vi "gums_measureLoop.vi"(0 "File Name":path=path "D:/users/test.dat", 1 "SaveDataQuery":bool=TRUE, 2 "Gain Cluster 2":T3={"Vsd"="Gate", "I 2probe 2"="Gate", "Vxy"="Gate", "Vxx"="Gate", "I leak BG"="Gate", "I leak TG"="Gate", "I Gain 1"=1000000.0, "V Gain 1"=1.0, "conversion factor BG"=1.0, "Vin / Vout 1"=1.0, "V Gain 2"=1.0, "Vin / Vout 2"=1.0, "V Gain 3"=1.0, "Vin / Vout 3"=1.0, "I Gain 2"=1000000.0, "I Gain 3"=1000000.0, "V BG"="Gate", "V TG"="Gate", "conversion factor TG"=1.0, "Vin / Vout 4"=1.0, "Vin / Vout 5"=1.0, "Manual Gain 1"=1.0, "Manual Gain 2"=1.0, "Manual Gain 3"=1.0} {"conversion factor TG" items=["1 V/V"=1.0, "4 V/V"=4.0, "15 V/V"=15.0, "30 V/V"=30.0, "45 V/V"=45.0]; "I Gain 3" items=["1"=1.0, "10"=10.0, "100"=100.0, "1K"=1000.0, "10K"=10000.0, "100K"=100000.0, "1M"=1000000.0, "10M"=10000000.0, "100M"=100000000.0, "1G"=1000000000.0]; "I Gain 2" items=["1"=1.0, "10"=10.0, "100"=100.0, "1K"=1000.0, "10K"=10000.0, "100K"=100000.0, "1M"=1000000.0, "10M"=10000000.0, "100M"=100000000.0, "1G"=1000000000.0]; "V Gain 3" items=["1"=1.0, "10"=10.0, "100"=100.0, "1K"=1000.0, "10K"=10000.0]; "V Gain 2" items=["1"=1.0, "10"=10.0, "100"=100.0, "1K"=1000.0, "10K"=10000.0]; "conversion factor BG" items=["1 V/V"=1.0, "4 V/V"=4.0, "15 V/V"=15.0, "30 V/V"=30.0, "45 V/V"=45.0]; "V Gain 1" items=["1"=1.0, "10"=10.0, "100"=100.0, "1K"=1000.0, "10K"=10000.0]; "I Gain 1" items=["1"=1.0, "10"=10.0, "100"=100.0, "1K"=1000.0, "10K"=10000.0, "100K"=100000.0, "1M"=1000000.0, "10M"=10000000.0, "100M"=100000000.0, "1G"=1000000000.0]}, 3 "Refresh Rate [ms]":i32=1000 min=0, 4 "Device Cluster":T4={"K2400 1"="", "K2400_1"=FALSE, "K2400 2"="", "K2400_2"=FALSE, "Lockin1"="", "Lockin1 present"=FALSE, "Lockin2"="", "Lockin2 present"=FALSE, "TIC"="", "Tcontrol"="OFF", "DMM1"="", "DMM1"=FALSE, "DMM2"="", "DMM2"=FALSE, "DAC"="", "DAC present"=FALSE, "DAC number 1"=0, "Bfield query"=FALSE, "Wvlen query"=FALSE, "ITC signal"={"ITC"=0, "Signal"=enum."Sensor 1"}, "DAC number 2"=0}) -> ()   [LabVIEW 2011]
uses:
  gumLV8p2/D/Labviewsoft/transport/GUMS/Kelvinox drivers/ITCAPPS - Copie.LLB/ITCSignal.ctl
  gumLV8p2/D/Labviewsoft/transport/GUMS/Kelvinox drivers/ITCAPPS - Copie.LLB/ITCSignals.ctl
  stopButton.vi
  DAC/DACreadglobal.vi
  Tglobalvar.vi
  monochromatorcontrol/perHandlemonochromator.vi
  users/nicolas/PHySpec-SDK-1.0.0/Labview-example/libPhyspec/libPhyspec.lvlib
panel:
  out "DAC 2 V [V]":dbl=1916.0
  out "DAC 2 array":dbl[](array[numeric])
  out "DAC number 2":u8=2 min=1 max=8
  out "Formula4Array":dbl[](array[numeric]) format="%.2f"
  out "Formula3Array":dbl[](array[numeric]) format="%.2f"
  out "Formula2Array":dbl[](array[numeric]) format="%.2f"
  in  "Formula 4":string
  in  "Formula 3":string
  in  "Formula 2":string
  out "Formula1Array":dbl[](array[numeric]) format="%.2f"
  in  "Formula 1":string
  out "Rxy Array":dbl[](array[numeric])
  out "ITC signal":T1={"ITC"=0, "Signal"=enum."Sensor 1"}
  in  "Fig3 Y scale 2":string(combo)="0"
  in  "Y-Axis 4":string(combo)="Gate"
  in  "X-Axis 4":string(combo)="Gate"
  out "Isd 4":cluster{"Bg":dbl[], "V_4probe":dbl[]}(graph)
  in  "Fig3 Y scale":string(combo)="0"
  in  "Y-Axis 3":string(combo)="Gate"
  in  "X-Axis 3":string(combo)="Gate"
  in  "Fig1 Y scale":string(combo)="0"
  in  "Fig2 Y scale":string(combo)="0"
  out "Fig 2":cluster{"Bg":dbl[], "V_4probe":dbl[]}(graph)
  in  "Y-Axis 1":string(combo)="Gate"
  in  "X-Axis 1":string(combo)="Gate"
  out "R4probe array":dbl[](array[numeric])
  out "R2probe array":dbl[](array[numeric])
  out "Itg array":dbl[](array[numeric])
  out "Ibg array":dbl[](array[numeric])
  out "Vxy array":dbl[](array[numeric])
  out "Vxx array":dbl[](array[numeric])
  out "Isd array":dbl[](array[numeric])
  out "Vsd array":dbl[](array[numeric])
  out "Vtg array":dbl[](array[numeric])
  out "Vbg array":dbl[](array[numeric])
  out "R 4probe [kOhm]":dbl=1916.0
  out "V_topgate [V]":dbl=1916.0
  out "V_backgate [V]":dbl=1916.0
  out "Vxy [V]":dbl=1916.0
  out "Vxx [V]":dbl=1916.0
  out "R 2probe [kOhm]":dbl=1916.0
  out "I Leak TG[nA]":dbl=1916.0
  out "I Leak BG [nA]":dbl=1916.0
  out "I 2probe [nA]":dbl=1916.0
  out "Vsd [V]":dbl=1916.0
  out "signal cluster":T5
  out "SetIntr Cluster":cluster{dbl, dbl, dbl, dbl, dbl}
  in  "Sensitivity Lockin2":T6(ring)
  in  "Sensitivity Lockin1":T6(ring)
  out "Wavelength array":dbl[](array[numeric])
  out "Wavelength [nm]":dbl=1916.0
  out "Wvlen query":bool
  out "refnum out":refnum<file>
  in  "Y-Axis 2":string(combo)="Gate"
  in  "X-Axis 2":string(combo)="Gate"
  out "DAC number 1":u8=2 min=1 max=8
  out "I K2400 01":dbl[](array[numeric])
  out "I K2400 02":dbl[](array[numeric])
  out "Voltage DMM2":dbl[](array[numeric])
  out "Voltage DMM1":dbl[](array[numeric])
  out "B":dbl[](array[numeric])
  out "Lockin2 X":dbl[](array[numeric])
  out "Lockin2 Y":dbl[](array[numeric])
  out "Lockin1 X":dbl[](array[numeric])
  out "B [T]":dbl=1916.0
  out "T [K]":dbl=1916.0
  out "Bfield query":bool
  out "I K2400_2 [A]":dbl=1916.0
  out "Lockin2 Y [V]":dbl=1916.0
  out "Lockin2 X [V]":dbl=1916.0
  out "V DMM2 [V]":dbl=1916.0
  out "V DMM1 [V]":dbl=1916.0
  out "I K2400_1 [A]":dbl=1916.0
  out "Lockin1 Y [V]":dbl=1916.0
  out "Lockin1 X [V]":dbl=1916.0
  out "Lockin1 Ampl [V]":dbl=1916.0
  out "K2400 1 [V]":dbl=1916.0
  out "K2400 2 [V]":dbl=1916.0
  out "DAC 1 V [V]":dbl=1916.0
  out "DAC present":bool
  out "K2400_2":bool
  out "K2400 2":refnum<visa-resource-name>="GPIB0::11::INSTR"
  out "DAC":refnum<visa-resource-name>="GPIB0::11::INSTR"
  out "DMM2":bool
  out "DMM1":bool
  out "Tcontrol":string
  out "Lockin2 present":bool
  out "Lockin1 present":bool
  out "K2400_1":bool
  out "DMM1":refnum<visa-resource-name>="GPIB0::11::INSTR"
  out "DMM2":refnum<visa-resource-name>="GPIB0::11::INSTR"
  out "TIC":refnum<visa-resource-name>="GPIB0::11::INSTR"
  out "Lockin2":refnum<visa-resource-name>="GPIB0::11::INSTR"
  out "Lockin1":refnum<visa-resource-name>="GPIB0::11::INSTR"
  out "K2400 1":refnum<visa-resource-name>="GPIB0::11::INSTR"
  out "Isd":cluster{"Bg":dbl[], "V_4probe":dbl[]}(graph)
  out "Isd 3":cluster{"Bg":dbl[], "V_4probe":dbl[]}(graph)
  out "stopMainLoop":bool
  out "V K2400_01 array":dbl[](array[numeric])
  out "Lockin1 Y":dbl[](array[numeric])
  out "DAC 1 array":dbl[](array[numeric])
  out "V K2400_02 array":dbl[](array[numeric])
  out "T":dbl[](array[numeric])
  out "Time":dbl[](array[numeric])
  out "Time [s]":dbl=1916.0
  in  "stop":bool
  # "Current run values"
  # "Magnetic Field"
  # "Wavelength"
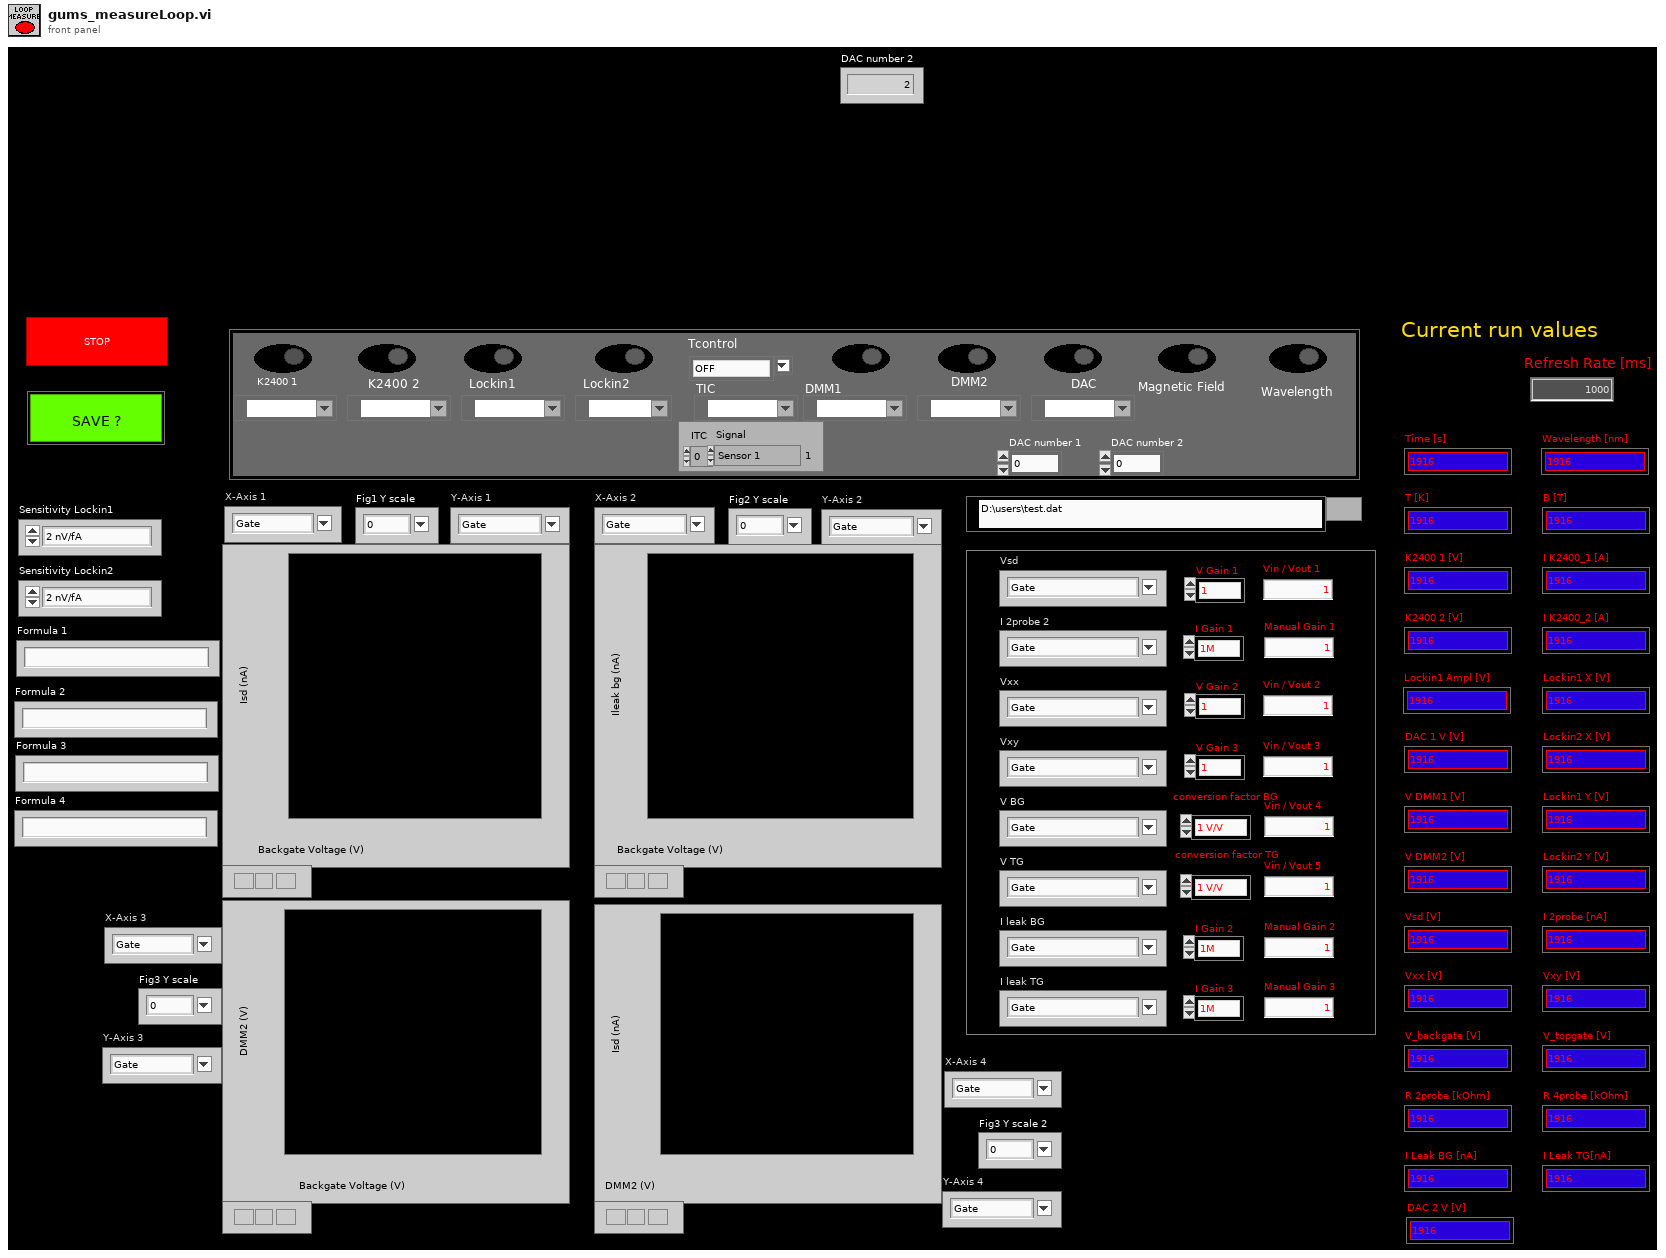
[diagram p1: front panel]
types:
  T1 = typedef "ITCSignal.ctl" = cluster{"ITC":u16, "Signal":T2}
  T2 = typedef "ITCSignals.ctl" = enum16{"Setpoint", "Sensor 1", "Sensor 2", "Sensor 3", "Needle Valve %", "Heater %"}
  T3 = cluster{"Vsd":string, "I 2probe 2":string, "Vxy":string, "Vxx":string, "I leak BG":string, "I leak TG":string, "I Gain 1":dbl, "V Gain 1":dbl, "conversion factor BG":dbl, "Vin / Vout 1":dbl, "V Gain 2":dbl, "Vin / Vout 2":dbl, "V Gain 3":dbl, "Vin / Vout 3":dbl, "I Gain 2":dbl, "I Gain 3":dbl, "V BG":string, "V TG":string, "conversion factor TG":dbl, "Vin / Vout 4":dbl, "Vin / Vout 5":dbl, "Manual Gain 1":dbl, "Manual Gain 2":dbl, "Manual Gain 3":dbl}
  T4 = cluster{"K2400 1":refnum<visa-resource-name>, "K2400_1":bool, "K2400 2":refnum<visa-resource-name>, "K2400_2":bool, "Lockin1":refnum<visa-resource-name>, "Lockin1 present":bool, "Lockin2":refnum<visa-resource-name>, "Lockin2 present":bool, "TIC":refnum<visa-resource-name>, "Tcontrol":string, "DMM1":refnum<visa-resource-name>, "DMM1":bool, "DMM2":refnum<visa-resource-name>, "DMM2":bool, "DAC":refnum<visa-resource-name>, "DAC present":bool, "DAC number 1":u8, "Bfield query":bool, "Wvlen query":bool, "ITC signal":T1, "DAC number 2":u8}
  T5 = cluster{"Output X":dbl, "Output X":dbl, "Voltage output":dbl, "Voltage output":dbl, dbl, dbl}
  T6 = enum16{"2 nV/fA", "5 nV/fA", "10 nV/fA", "20 nV/fA", "50 nV/fA", "100 nV/fA", "200 nV/fA", "500 nV/fA", "1 uV/pA", "2 uV/pA", "5 uV/pA", "10 uV/pA", "20 uV/pA", "50 uV/pA", "100 uV/pA", "200 uV/pA", "500 uV/pA", "1 mV/nA", "2 mV/nA", "5 mV/nA", "10 mV/nA", "20 mV/nA", "50 mV/nA", "100 mV/nA", "200 mV/nA", "500 mV/nA", "1 V/uA"}
  T7 = cluster{"Formula4Array":dbl[], "Formula4Array":dbl[]}
  T8 = cluster{"Output X":dbl, "Output X":dbl, "Voltage output":dbl, "Voltage output":dbl, "I K2400_1 [A]":dbl, "I K2400_2 [A]":dbl}
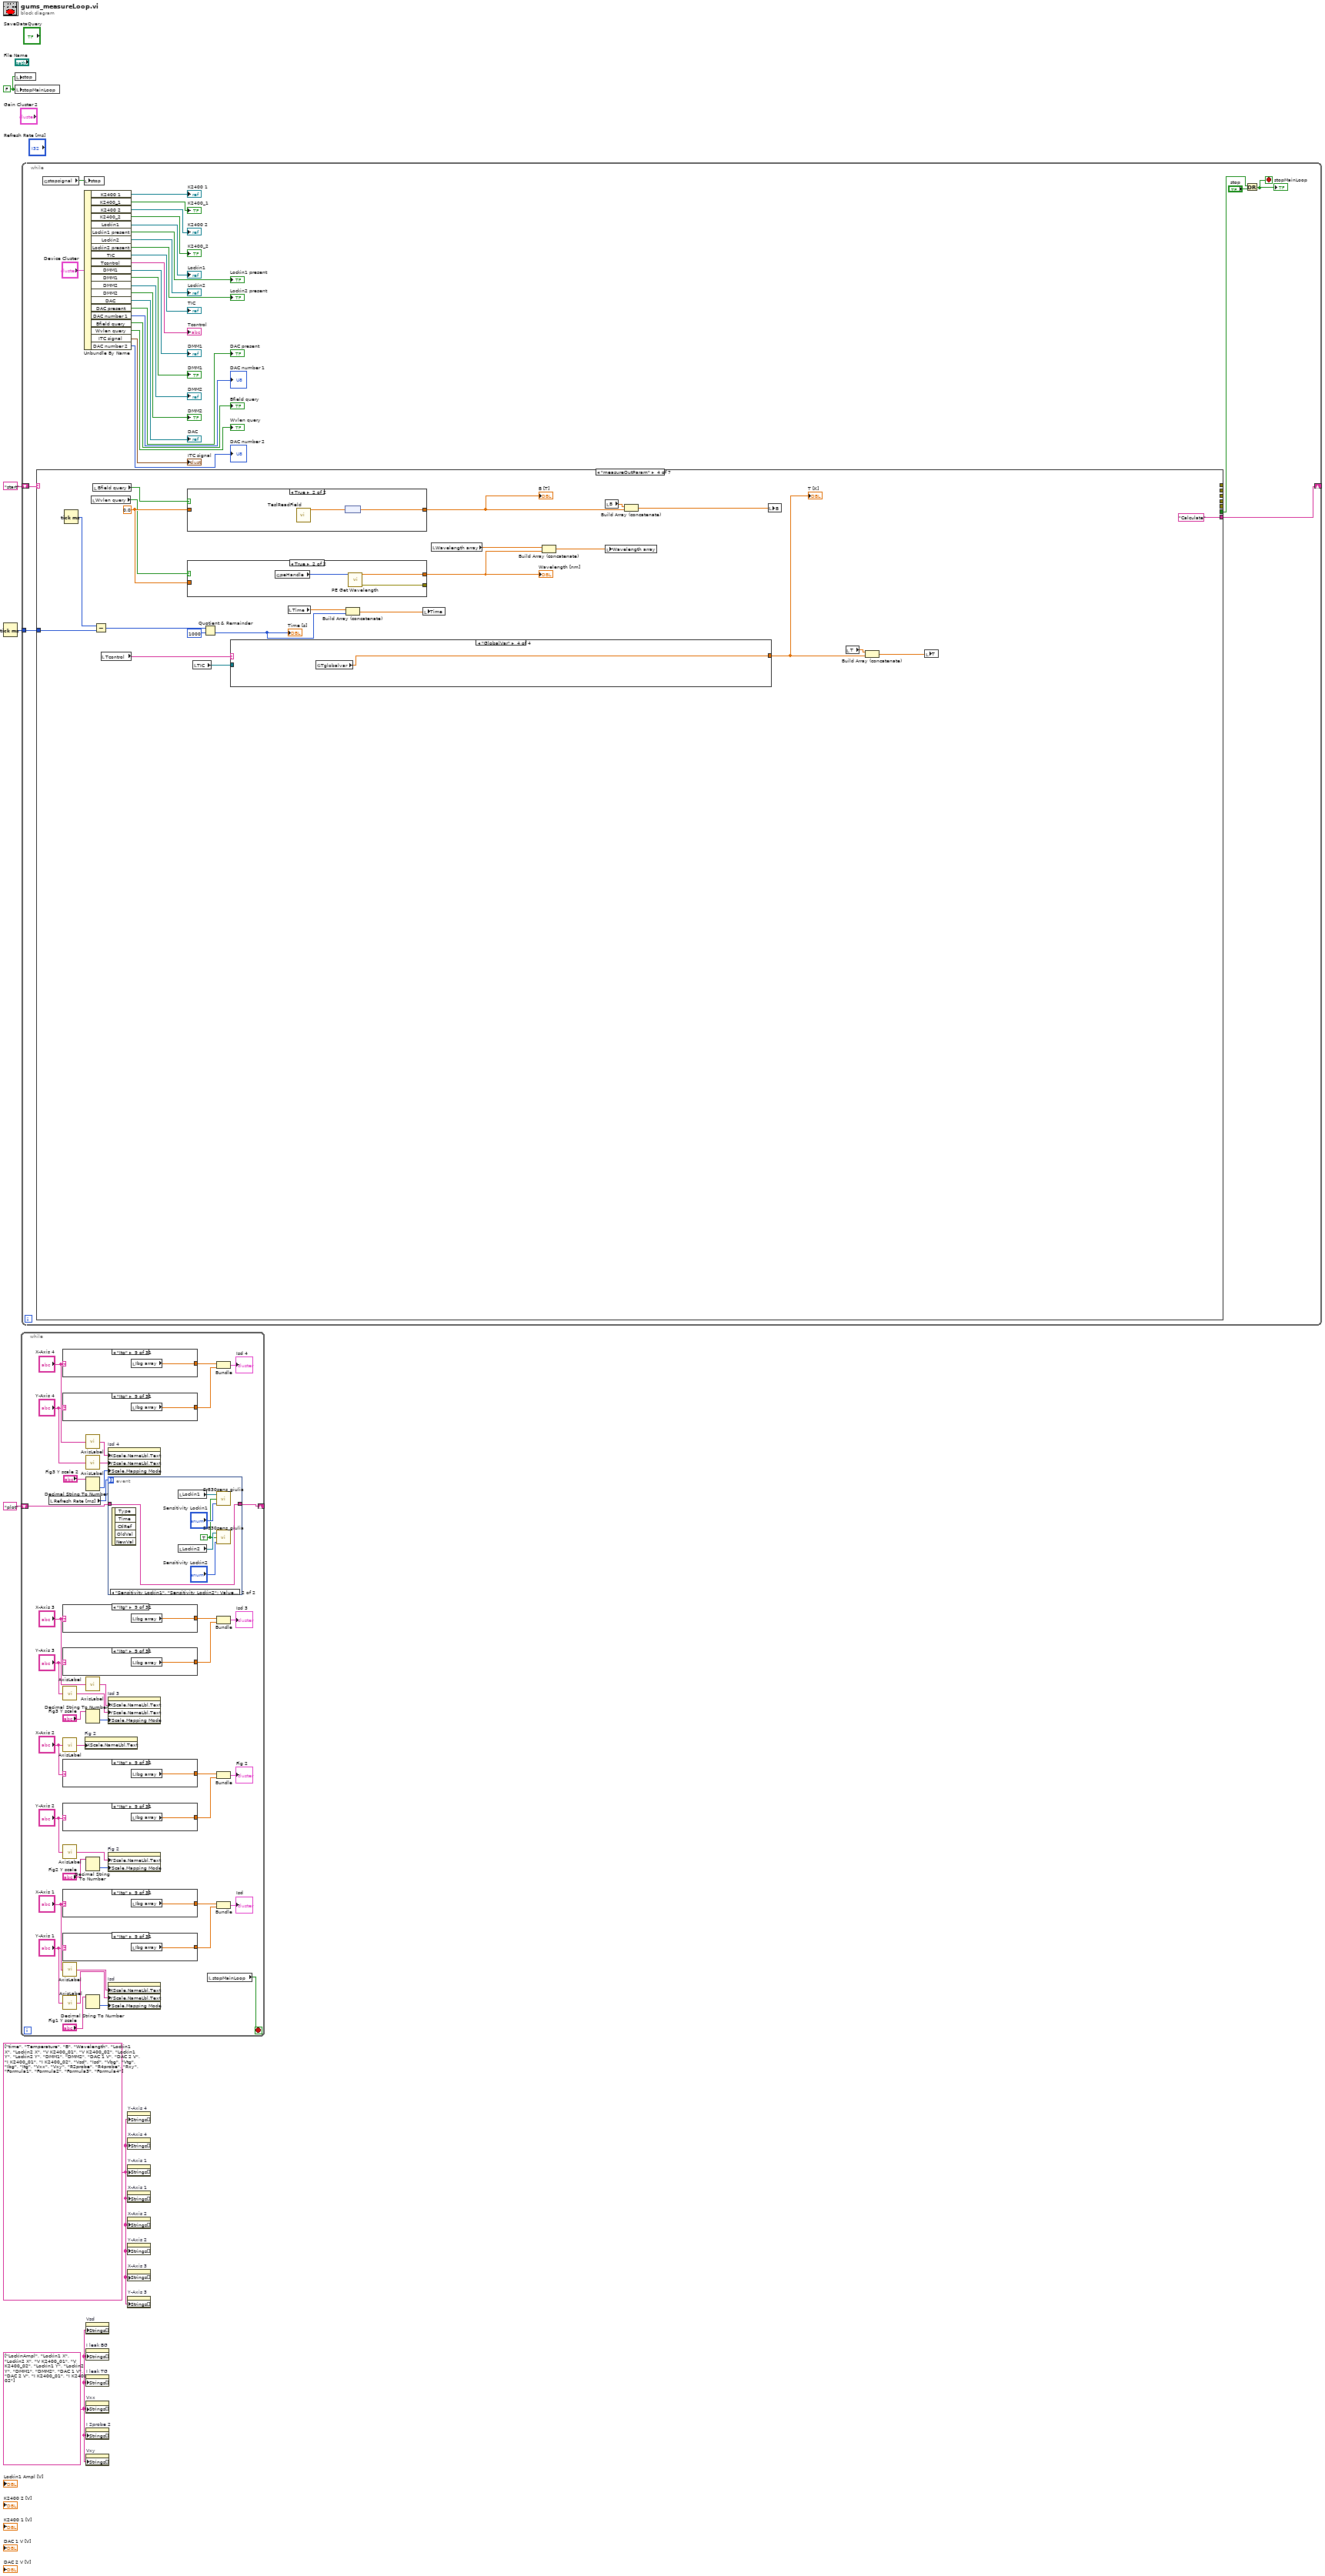
[diagram p0: block diagram]
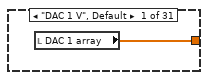
[diagram p2: hidden frame]
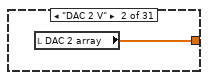
[diagram p3: hidden frame]
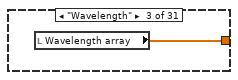
[diagram p4: hidden frame]
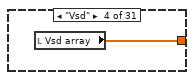
[diagram p5: hidden frame]
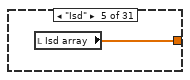
[diagram p6: hidden frame]
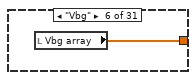
[diagram p7: hidden frame]
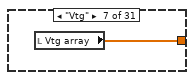
[diagram p8: hidden frame]
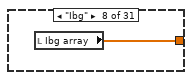
[diagram p9: hidden frame]
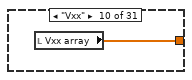
[diagram p10: hidden frame]
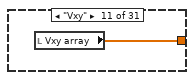
[diagram p11: hidden frame]
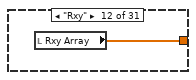
[diagram p12: hidden frame]
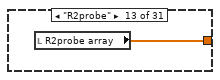
[diagram p13: hidden frame]
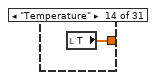
[diagram p14: hidden frame]
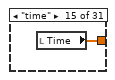
[diagram p15: hidden frame]
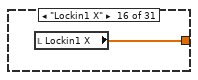
[diagram p16: hidden frame]
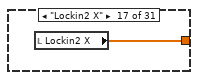
[diagram p17: hidden frame]
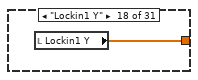
[diagram p18: hidden frame]
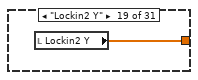
[diagram p19: hidden frame]
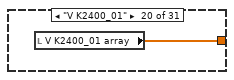
[diagram p20: hidden frame]
diagram:
  w1 = string[] ["time", "Temperature", "B", "Wavelength", "Lockin1 X", "Lockin2 X", "V K2400_01", "V K2400_02", "Lockin1 Y", "Lockin2 Y", "DMM1", "DMM2", "DAC 1 V", "DAC 2 V", "I K2400_01", "I K2400_02", "Vsd", "Isd", "Vbg", "Vtg", "Ibg", "Itg", "Vxx", "Vxy", "R2probe", "R4probe", "Rxy", "Formula1", "Formula2", "Formula3", "Formula4"] ("Axis select")
  w3 = string[] ["LockinAmpl", "Lockin1 X", "Lockin2 X", "V K2400_01", "V K2400_02", "Lockin1 Y", "Lockin2 Y", "DMM1", "DMM2", "DAC 1 V", "DAC 2 V", "I K2400_01", "I K2400_02"] ("Strings []")
  w4 = FALSE ("stop")
  n1 = Tick Count (ms)() -> (millisecond timer value=w5:u32)
  n2 = local write "stop"(w4) -> ()
  n3 = local write "stopMainLoop"(w4) -> ()
  n4 = while {
    shift-right: [w43] -> _
    shift-left: "plot" -> [w44]
    stop <- w45 stop-if-true
    n5 = local read "Refresh Rate [ms]"() -> (w40:i32)
    n6 = case shown="\"Itg\"" "X-Axis 4" {
      tunnel: [w202 w203 w204 w205 w206 w207 w208 w209 w210 w211 w212 w213 w214 w215 w216 w217 w218 w219 w220 w221 w222 w223 w224 w225 w226 w227 w228 w229 w230 w231 w232] -> w18
      frame "DAC 1 V", Default {
        n7 = local read "DAC 1 array"() -> (w202:dbl[])
      }
      frame "DAC 2 V" {
        n8 = local read "DAC 2 array"() -> (w203:dbl[])
      }
      frame "Wavelength" {
        n9 = local read "Wavelength array"() -> (w204:dbl[])
      }
      frame "Vsd" {
        n10 = local read "Vsd array"() -> (w205:dbl[])
      }
      frame "Isd" {
        n11 = local read "Isd array"() -> (w206:dbl[])
      }
      frame "Vbg" {
        n12 = local read "Vbg array"() -> (w207:dbl[])
      }
      frame "Vtg" {
        n13 = local read "Vtg array"() -> (w208:dbl[])
      }
      frame "Ibg" {
        n14 = local read "Ibg array"() -> (w209:dbl[])
      }
      frame "Itg" {
        n15 = local read "Ibg array"() -> (w210:dbl[])
      }
      frame "Vxx" {
        n16 = local read "Vxx array"() -> (w211:dbl[])
      }
      frame "Vxy" {
        n17 = local read "Vxy array"() -> (w212:dbl[])
      }
      frame "Rxy" {
        n18 = local read "Rxy Array"() -> (w213:dbl[])
      }
      frame "R2probe" {
        n19 = local read "R2probe array"() -> (w214:dbl[])
      }
      frame "Temperature" {
        n20 = local read "T"() -> (w215:dbl[])
      }
      frame "time" {
        n21 = local read "Time"() -> (w216:dbl[])
      }
      frame "Lockin1 X" {
        n22 = local read "Lockin1 X"() -> (w217:dbl[])
      }
      frame "Lockin2 X" {
        n23 = local read "Lockin2 X"() -> (w218:dbl[])
      }
      frame "Lockin1 Y" {
        n24 = local read "Lockin1 Y"() -> (w219:dbl[])
      }
      frame "Lockin2 Y" {
        n25 = local read "Lockin2 Y"() -> (w220:dbl[])
      }
      frame "V K2400_01" {
        n26 = local read "V K2400_01 array"() -> (w221:dbl[])
      }
      frame "V K2400_02" {
        n27 = local read "V K2400_02 array"() -> (w222:dbl[])
      }
      frame "I K2400_01" {
        n28 = local read "I K2400 01"() -> (w223:dbl[])
      }
      frame "I K2400_02" {
        n29 = local read "I K2400 02"() -> (w224:dbl[])
      }
      frame "DMM1" {
        n30 = local read "Voltage DMM1"() -> (w225:dbl[])
      }
      frame "DMM2" {
        n31 = local read "Voltage DMM2"() -> (w226:dbl[])
      }
      frame "B" {
        n32 = local read "B"() -> (w227:dbl[])
      }
      frame "R4probe" {
        n33 = local read "R4probe array"() -> (w228:dbl[])
      }
      frame "Formula1" {
        n34 = local read "Formula1Array"() -> (w229:dbl[])
      }
      frame "Formula2" {
        n35 = local read "Formula2Array"() -> (w230:dbl[])
      }
      frame "Formula3" {
        n36 = local read "Formula3Array"() -> (w231:dbl[])
      }
      frame "Formula4" {
        n37 = local read "Formula4Array"() -> (w232:dbl[])
      }
    }
    n38 = case shown="\"Itg\"" "Y-Axis 4" {
      tunnel: [w171 w172 w173 w174 w175 w176 w177 w178 w179 w180 w181 w182 w183 w184 w185 w186 w187 w188 w189 w190 w191 w192 w193 w194 w195 w196 w197 w198 w199 w200 w201] -> w16
      frame "DAC 1 V", Default {
        n39 = local read "DAC 1 array"() -> (w171:dbl[])
      }
      frame "DAC 2 V" {
        n40 = local read "DAC 2 array"() -> (w172:dbl[])
      }
      frame "Wavelength" {
        n41 = local read "Wavelength array"() -> (w173:dbl[])
      }
      frame "Vsd" {
        n42 = local read "Vsd array"() -> (w174:dbl[])
      }
      frame "Isd" {
        n43 = local read "Isd array"() -> (w175:dbl[])
      }
      frame "Vbg" {
        n44 = local read "Vbg array"() -> (w176:dbl[])
      }
      frame "Vtg" {
        n45 = local read "Vtg array"() -> (w177:dbl[])
      }
      frame "Ibg" {
        n46 = local read "Ibg array"() -> (w178:dbl[])
      }
      frame "Itg" {
        n47 = local read "Ibg array"() -> (w179:dbl[])
      }
      frame "Vxx" {
        n48 = local read "Vxx array"() -> (w180:dbl[])
      }
      frame "Vxy" {
        n49 = local read "Vxy array"() -> (w181:dbl[])
      }
      frame "Rxy" {
        n50 = local read "Rxy Array"() -> (w182:dbl[])
      }
      frame "R2probe" {
        n51 = local read "R2probe array"() -> (w183:dbl[])
      }
      frame "Temperature" {
        n52 = local read "T"() -> (w184:dbl[])
      }
      frame "time" {
        n53 = local read "Time"() -> (w185:dbl[])
      }
      frame "Lockin1 X" {
        n54 = local read "Lockin1 X"() -> (w186:dbl[])
      }
      frame "Lockin2 X" {
        n55 = local read "Lockin2 X"() -> (w187:dbl[])
      }
      frame "Lockin1 Y" {
        n56 = local read "Lockin1 Y"() -> (w188:dbl[])
      }
      frame "Lockin2 Y" {
        n57 = local read "Lockin2 Y"() -> (w189:dbl[])
      }
      frame "V K2400_01" {
        n58 = local read "V K2400_01 array"() -> (w190:dbl[])
      }
      frame "V K2400_02" {
        n59 = local read "V K2400_02 array"() -> (w191:dbl[])
      }
      frame "I K2400_01" {
        n60 = local read "I K2400 01"() -> (w192:dbl[])
      }
      frame "I K2400_02" {
        n61 = local read "I K2400 02"() -> (w193:dbl[])
      }
      frame "DMM1" {
        n62 = local read "Voltage DMM1"() -> (w194:dbl[])
      }
      frame "DMM2" {
        n63 = local read "Voltage DMM2"() -> (w195:dbl[])
      }
      frame "B" {
        n64 = local read "B"() -> (w196:dbl[])
      }
      frame "R4probe" {
        n65 = local read "R4probe array"() -> (w197:dbl[])
      }
      frame "Formula1" {
        n66 = local read "Formula1Array"() -> (w198:dbl[])
      }
      frame "Formula2" {
        n67 = local read "Formula2Array"() -> (w199:dbl[])
      }
      frame "Formula3" {
        n68 = local read "Formula3Array"() -> (w200:dbl[])
      }
      frame "Formula4" {
        n69 = local read "Formula4Array"() -> (w201:dbl[])
      }
    }
    n70 = case shown="\"Itg\"" "X-Axis 3" {
      tunnel: [w140 w141 w142 w143 w144 w145 w146 w147 w148 w149 w150 w151 w152 w153 w154 w155 w156 w157 w158 w159 w160 w161 w162 w163 w164 w165 w166 w167 w168 w169 w170] -> w13
      frame "DAC 1 V", Default {
        n71 = local read "DAC 1 array"() -> (w140:dbl[])
      }
      frame "DAC 2 V" {
        n72 = local read "DAC 2 array"() -> (w141:dbl[])
      }
      frame "Wavelength" {
        n73 = local read "Wavelength array"() -> (w142:dbl[])
      }
      frame "Vsd" {
        n74 = local read "Vsd array"() -> (w143:dbl[])
      }
      frame "Isd" {
        n75 = local read "Isd array"() -> (w144:dbl[])
      }
      frame "Vbg" {
        n76 = local read "Vbg array"() -> (w145:dbl[])
      }
      frame "Vtg" {
        n77 = local read "Vtg array"() -> (w146:dbl[])
      }
      frame "Ibg" {
        n78 = local read "Ibg array"() -> (w147:dbl[])
      }
      frame "Itg" {
        n79 = local read "Ibg array"() -> (w148:dbl[])
      }
      frame "Vxx" {
        n80 = local read "Vxx array"() -> (w149:dbl[])
      }
      frame "Vxy" {
        n81 = local read "Vxy array"() -> (w150:dbl[])
      }
      frame "Rxy" {
        n82 = local read "Rxy Array"() -> (w151:dbl[])
      }
      frame "R2probe" {
        n83 = local read "R2probe array"() -> (w152:dbl[])
      }
      frame "Temperature" {
        n84 = local read "T"() -> (w153:dbl[])
      }
      frame "time" {
        n85 = local read "Time"() -> (w154:dbl[])
      }
      frame "Lockin1 X" {
        n86 = local read "Lockin1 X"() -> (w155:dbl[])
      }
      frame "Lockin2 X" {
        n87 = local read "Lockin2 X"() -> (w156:dbl[])
      }
      frame "Lockin1 Y" {
        n88 = local read "Lockin1 Y"() -> (w157:dbl[])
      }
      frame "Lockin2 Y" {
        n89 = local read "Lockin2 Y"() -> (w158:dbl[])
      }
      frame "V K2400_01" {
        n90 = local read "V K2400_01 array"() -> (w159:dbl[])
      }
      frame "V K2400_02" {
        n91 = local read "V K2400_02 array"() -> (w160:dbl[])
      }
      frame "I K2400_01" {
        n92 = local read "I K2400 01"() -> (w161:dbl[])
      }
      frame "I K2400_02" {
        n93 = local read "I K2400 02"() -> (w162:dbl[])
      }
      frame "DMM1" {
        n94 = local read "Voltage DMM1"() -> (w163:dbl[])
      }
      frame "DMM2" {
        n95 = local read "Voltage DMM2"() -> (w164:dbl[])
      }
      frame "B" {
        n96 = local read "B"() -> (w165:dbl[])
      }
      frame "R4probe" {
        n97 = local read "R4probe array"() -> (w166:dbl[])
      }
      frame "Formula1" {
        n98 = local read "Formula1Array"() -> (w167:dbl[])
      }
      frame "Formula2" {
        n99 = local read "Formula2Array"() -> (w168:dbl[])
      }
      frame "Formula3" {
        n100 = local read "Formula3Array"() -> (w169:dbl[])
      }
      frame "Formula4" {
        n101 = local read "Formula4Array"() -> (w170:dbl[])
      }
    }
    n102 = case shown="\"Itg\"" "Y-Axis 3" {
      tunnel: [w109 w110 w111 w112 w113 w114 w115 w116 w117 w118 w119 w120 w121 w122 w123 w124 w125 w126 w127 w128 w129 w130 w131 w132 w133 w134 w135 w136 w137 w138 w139] -> w14
      frame "DAC 1 V", Default {
        n103 = local read "DAC 1 array"() -> (w109:dbl[])
      }
      frame "DAC 2 V" {
        n104 = local read "DAC 2 array"() -> (w110:dbl[])
      }
      frame "Wavelength" {
        n105 = local read "Wavelength array"() -> (w111:dbl[])
      }
      frame "Vsd" {
        n106 = local read "Vsd array"() -> (w112:dbl[])
      }
      frame "Isd" {
        n107 = local read "Isd array"() -> (w113:dbl[])
      }
      frame "Vbg" {
        n108 = local read "Vbg array"() -> (w114:dbl[])
      }
      frame "Vtg" {
        n109 = local read "Vtg array"() -> (w115:dbl[])
      }
      frame "Ibg" {
        n110 = local read "Ibg array"() -> (w116:dbl[])
      }
      frame "Itg" {
        n111 = local read "Ibg array"() -> (w117:dbl[])
      }
      frame "Vxx" {
        n112 = local read "Vxx array"() -> (w118:dbl[])
      }
      frame "Vxy" {
        n113 = local read "Vxy array"() -> (w119:dbl[])
      }
      frame "Rxy" {
        n114 = local read "Rxy Array"() -> (w120:dbl[])
      }
      frame "R2probe" {
        n115 = local read "R2probe array"() -> (w121:dbl[])
      }
      frame "Temperature" {
        n116 = local read "T"() -> (w122:dbl[])
      }
      frame "time" {
        n117 = local read "Time"() -> (w123:dbl[])
      }
      frame "Lockin1 X" {
        n118 = local read "Lockin1 X"() -> (w124:dbl[])
      }
      frame "Lockin2 X" {
        n119 = local read "Lockin2 X"() -> (w125:dbl[])
      }
      frame "Lockin1 Y" {
        n120 = local read "Lockin1 Y"() -> (w126:dbl[])
      }
      frame "Lockin2 Y" {
        n121 = local read "Lockin2 Y"() -> (w127:dbl[])
      }
      frame "V K2400_01" {
        n122 = local read "V K2400_01 array"() -> (w128:dbl[])
      }
      frame "V K2400_02" {
        n123 = local read "V K2400_02 array"() -> (w129:dbl[])
      }
      frame "I K2400_01" {
        n124 = local read "I K2400 01"() -> (w130:dbl[])
      }
      frame "I K2400_02" {
        n125 = local read "I K2400 02"() -> (w131:dbl[])
      }
      frame "DMM1" {
        n126 = local read "Voltage DMM1"() -> (w132:dbl[])
      }
      frame "DMM2" {
        n127 = local read "Voltage DMM2"() -> (w133:dbl[])
      }
      frame "B" {
        n128 = local read "B"() -> (w134:dbl[])
      }
      frame "R4probe" {
        n129 = local read "R4probe array"() -> (w135:dbl[])
      }
      frame "Formula1" {
        n130 = local read "Formula1Array"() -> (w136:dbl[])
      }
      frame "Formula2" {
        n131 = local read "Formula2Array"() -> (w137:dbl[])
      }
      frame "Formula3" {
        n132 = local read "Formula3Array"() -> (w138:dbl[])
      }
      frame "Formula4" {
        n133 = local read "Formula4Array"() -> (w139:dbl[])
      }
    }
    n134 = call "AxisLabel.vi"("Axis"="Y-Axis 3") -> ("X Scale.Name Label.Text"=w29:string)
    n135 = call "AxisLabel.vi"("Axis"="X-Axis 2") -> ("X Scale.Name Label.Text"=w41:string)
    n136 = case shown="\"Itg\"" "X-Axis 2" {
      tunnel: [w47 w48 w49 w50 w51 w52 w53 w54 w55 w56 w57 w58 w59 w60 w61 w62 w63 w64 w65 w66 w67 w68 w69 w70 w71 w72 w73 w74 w75 w76 w77] -> w8
      frame "DAC 1 V", Default {
        n137 = local read "DAC 1 array"() -> (w47:dbl[])
      }
      frame "DAC 2 V" {
        n138 = local read "DAC 2 array"() -> (w48:dbl[])
      }
      frame "Wavelength" {
        n139 = local read "Wavelength array"() -> (w49:dbl[])
      }
      frame "Vsd" {
        n140 = local read "Vsd array"() -> (w50:dbl[])
      }
      frame "Isd" {
        n141 = local read "Isd array"() -> (w51:dbl[])
      }
      frame "Vbg" {
        n142 = local read "Vbg array"() -> (w52:dbl[])
      }
      frame "Vtg" {
        n143 = local read "Vtg array"() -> (w53:dbl[])
      }
      frame "Ibg" {
        n144 = local read "Ibg array"() -> (w54:dbl[])
      }
      frame "Itg" {
        n145 = local read "Ibg array"() -> (w55:dbl[])
      }
      frame "Vxx" {
        n146 = local read "Vxx array"() -> (w56:dbl[])
      }
      frame "Vxy" {
        n147 = local read "Vxy array"() -> (w57:dbl[])
      }
      frame "Rxy" {
        n148 = local read "Rxy Array"() -> (w58:dbl[])
      }
      frame "R2probe" {
        n149 = local read "R2probe array"() -> (w59:dbl[])
      }
      frame "Temperature" {
        n150 = local read "T"() -> (w60:dbl[])
      }
      frame "time" {
        n151 = local read "Time"() -> (w61:dbl[])
      }
      frame "Lockin1 X" {
        n152 = local read "Lockin1 X"() -> (w62:dbl[])
      }
      frame "Lockin2 X" {
        n153 = local read "Lockin2 X"() -> (w63:dbl[])
      }
      frame "Lockin1 Y" {
        n154 = local read "Lockin1 Y"() -> (w64:dbl[])
      }
      frame "Lockin2 Y" {
        n155 = local read "Lockin2 Y"() -> (w65:dbl[])
      }
      frame "V K2400_01" {
        n156 = local read "V K2400_01 array"() -> (w66:dbl[])
      }
      frame "V K2400_02" {
        n157 = local read "V K2400_02 array"() -> (w67:dbl[])
      }
      frame "I K2400_01" {
        n158 = local read "I K2400 01"() -> (w68:dbl[])
      }
      frame "I K2400_02" {
        n159 = local read "I K2400 02"() -> (w69:dbl[])
      }
      frame "DMM1" {
        n160 = local read "Voltage DMM1"() -> (w70:dbl[])
      }
      frame "DMM2" {
        n161 = local read "Voltage DMM2"() -> (w71:dbl[])
      }
      frame "B" {
        n162 = local read "B"() -> (w72:dbl[])
      }
      frame "R4probe" {
        n163 = local read "R4probe array"() -> (w73:dbl[])
      }
      frame "Formula1" {
        n164 = local read "Formula1Array"() -> (w74:dbl[])
      }
      frame "Formula2" {
        n165 = local read "Formula2Array"() -> (w75:dbl[])
      }
      frame "Formula3" {
        n166 = local read "Formula3Array"() -> (w76:dbl[])
      }
      frame "Formula4" {
        n167 = local read "Formula4Array"() -> (w77:dbl[])
      }
    }
    n168 = case shown="\"Itg\"" "Y-Axis 2" {
      tunnel: [w78 w79 w80 w81 w82 w83 w84 w85 w86 w87 w88 w89 w90 w91 w92 w93 w94 w95 w96 w97 w98 w99 w100 w101 w102 w103 w104 w105 w106 w107 w108] -> w9
      frame "DAC 1 V", Default {
        n169 = local read "DAC 1 array"() -> (w78:dbl[])
      }
      frame "DAC 2 V" {
        n170 = local read "DAC 2 array"() -> (w79:dbl[])
      }
      frame "Wavelength" {
        n171 = local read "Wavelength array"() -> (w80:dbl[])
      }
      frame "Vsd" {
        n172 = local read "Vsd array"() -> (w81:dbl[])
      }
      frame "Isd" {
        n173 = local read "Isd array"() -> (w82:dbl[])
      }
      frame "Vbg" {
        n174 = local read "Vbg array"() -> (w83:dbl[])
      }
      frame "Vtg" {
        n175 = local read "Vtg array"() -> (w84:dbl[])
      }
      frame "Ibg" {
        n176 = local read "Ibg array"() -> (w85:dbl[])
      }
      frame "Itg" {
        n177 = local read "Ibg array"() -> (w86:dbl[])
      }
      frame "Vxx" {
        n178 = local read "Vxx array"() -> (w87:dbl[])
      }
      frame "Vxy" {
        n179 = local read "Vxy array"() -> (w88:dbl[])
      }
      frame "Rxy" {
        n180 = local read "Rxy Array"() -> (w89:dbl[])
      }
      frame "R2probe" {
        n181 = local read "R2probe array"() -> (w90:dbl[])
      }
      frame "Temperature" {
        n182 = local read "T"() -> (w91:dbl[])
      }
      frame "time" {
        n183 = local read "Time"() -> (w92:dbl[])
      }
      frame "Lockin1 X" {
        n184 = local read "Lockin1 X"() -> (w93:dbl[])
      }
      frame "Lockin2 X" {
        n185 = local read "Lockin2 X"() -> (w94:dbl[])
      }
      frame "Lockin1 Y" {
        n186 = local read "Lockin1 Y"() -> (w95:dbl[])
      }
      frame "Lockin2 Y" {
        n187 = local read "Lockin2 Y"() -> (w96:dbl[])
      }
      frame "V K2400_01" {
        n188 = local read "V K2400_01 array"() -> (w97:dbl[])
      }
      frame "V K2400_02" {
        n189 = local read "V K2400_02 array"() -> (w98:dbl[])
      }
      frame "I K2400_01" {
        n190 = local read "I K2400 01"() -> (w99:dbl[])
      }
      frame "I K2400_02" {
        n191 = local read "I K2400 02"() -> (w100:dbl[])
      }
      frame "DMM1" {
        n192 = local read "Voltage DMM1"() -> (w101:dbl[])
      }
      frame "DMM2" {
        n193 = local read "Voltage DMM2"() -> (w102:dbl[])
      }
      frame "B" {
        n194 = local read "B"() -> (w103:dbl[])
      }
      frame "R4probe" {
        n195 = local read "R4probe array"() -> (w104:dbl[])
      }
      frame "Formula1" {
        n196 = local read "Formula1Array"() -> (w105:dbl[])
      }
      frame "Formula2" {
        n197 = local read "Formula2Array"() -> (w106:dbl[])
      }
      frame "Formula3" {
        n198 = local read "Formula3Array"() -> (w107:dbl[])
      }
      frame "Formula4" {
        n199 = local read "Formula4Array"() -> (w108:dbl[])
      }
    }
    n200 = call "AxisLabel.vi"("Axis"="Y-Axis 2") -> ("X Scale.Name Label.Text"=w42:string)
    n201 = case shown="\"Itg\"" "X-Axis 1" {
      tunnel: [w264 w265 w266 w267 w268 w269 w270 w271 w272 w273 w274 w275 w276 w277 w278 w279 w280 w281 w282 w283 w284 w285 w286 w287 w288 w289 w290 w291 w292 w293 w294] -> w22
      frame "DAC 1 V", Default {
        n202 = local read "DAC 1 array"() -> (w264:dbl[])
      }
      frame "DAC 2 V" {
        n203 = local read "DAC 2 array"() -> (w265:dbl[])
      }
      frame "Wavelength" {
        n204 = local read "Wavelength array"() -> (w266:dbl[])
      }
      frame "Vsd" {
        n205 = local read "Vsd array"() -> (w267:dbl[])
      }
      frame "Isd" {
        n206 = local read "Isd array"() -> (w268:dbl[])
      }
      frame "Vbg" {
        n207 = local read "Vbg array"() -> (w269:dbl[])
      }
      frame "Vtg" {
        n208 = local read "Vtg array"() -> (w270:dbl[])
      }
      frame "Ibg" {
        n209 = local read "Ibg array"() -> (w271:dbl[])
      }
      frame "Itg" {
        n210 = local read "Ibg array"() -> (w272:dbl[])
      }
      frame "Vxx" {
        n211 = local read "Vxx array"() -> (w273:dbl[])
      }
      frame "Vxy" {
        n212 = local read "Vxy array"() -> (w274:dbl[])
      }
      frame "Rxy" {
        n213 = local read "Rxy Array"() -> (w275:dbl[])
      }
      frame "R2probe" {
        n214 = local read "R2probe array"() -> (w276:dbl[])
      }
      frame "Temperature" {
        n215 = local read "T"() -> (w277:dbl[])
      }
      frame "time" {
        n216 = local read "Time"() -> (w278:dbl[])
      }
      frame "Lockin1 X" {
        n217 = local read "Lockin1 X"() -> (w279:dbl[])
      }
      frame "Lockin2 X" {
        n218 = local read "Lockin2 X"() -> (w280:dbl[])
      }
      frame "Lockin1 Y" {
        n219 = local read "Lockin1 Y"() -> (w281:dbl[])
      }
      frame "Lockin2 Y" {
        n220 = local read "Lockin2 Y"() -> (w282:dbl[])
      }
      frame "V K2400_01" {
        n221 = local read "V K2400_01 array"() -> (w283:dbl[])
      }
      frame "V K2400_02" {
        n222 = local read "V K2400_02 array"() -> (w284:dbl[])
      }
      frame "I K2400_01" {
        n223 = local read "I K2400 01"() -> (w285:dbl[])
      }
      frame "I K2400_02" {
        n224 = local read "I K2400 02"() -> (w286:dbl[])
      }
      frame "DMM1" {
        n225 = local read "Voltage DMM1"() -> (w287:dbl[])
      }
      frame "DMM2" {
        n226 = local read "Voltage DMM2"() -> (w288:dbl[])
      }
      frame "B" {
        n227 = local read "B"() -> (w289:dbl[])
      }
      frame "R4probe" {
        n228 = local read "R4probe array"() -> (w290:dbl[])
      }
      frame "Formula1" {
        n229 = local read "Formula1Array"() -> (w291:dbl[])
      }
      frame "Formula2" {
        n230 = local read "Formula2Array"() -> (w292:dbl[])
      }
      frame "Formula3" {
        n231 = local read "Formula3Array"() -> (w293:dbl[])
      }
      frame "Formula4" {
        n232 = local read "Formula4Array"() -> (w294:dbl[])
      }
    }
    n233 = case shown="\"Itg\"" "Y-Axis 1" {
      tunnel: [w233 w234 w235 w236 w237 w238 w239 w240 w241 w242 w243 w244 w245 w246 w247 w248 w249 w250 w251 w252 w253 w254 w255 w256 w257 w258 w259 w260 w261 w262 w263] -> w19
      frame "DAC 1 V", Default {
        n234 = local read "DAC 1 array"() -> (w233:dbl[])
      }
      frame "DAC 2 V" {
        n235 = local read "DAC 2 array"() -> (w234:dbl[])
      }
      frame "Wavelength" {
        n236 = local read "Wavelength array"() -> (w235:dbl[])
      }
      frame "Vsd" {
        n237 = local read "Vsd array"() -> (w236:dbl[])
      }
      frame "Isd" {
        n238 = local read "Isd array"() -> (w237:dbl[])
      }
      frame "Vbg" {
        n239 = local read "Vbg array"() -> (w238:dbl[])
      }
      frame "Vtg" {
        n240 = local read "Vtg array"() -> (w239:dbl[])
      }
      frame "Ibg" {
        n241 = local read "Ibg array"() -> (w240:dbl[])
      }
      frame "Itg" {
        n242 = local read "Ibg array"() -> (w241:dbl[])
      }
      frame "Vxx" {
        n243 = local read "Vxx array"() -> (w242:dbl[])
      }
      frame "Vxy" {
        n244 = local read "Vxy array"() -> (w243:dbl[])
      }
      frame "Rxy" {
        n245 = local read "Rxy Array"() -> (w244:dbl[])
      }
      frame "R2probe" {
        n246 = local read "R2probe array"() -> (w245:dbl[])
      }
      frame "Temperature" {
        n247 = local read "T"() -> (w246:dbl[])
      }
      frame "time" {
        n248 = local read "Time"() -> (w247:dbl[])
      }
      frame "Lockin1 X" {
        n249 = local read "Lockin1 X"() -> (w248:dbl[])
      }
      frame "Lockin2 X" {
        n250 = local read "Lockin2 X"() -> (w249:dbl[])
      }
      frame "Lockin1 Y" {
        n251 = local read "Lockin1 Y"() -> (w250:dbl[])
      }
      frame "Lockin2 Y" {
        n252 = local read "Lockin2 Y"() -> (w251:dbl[])
      }
      frame "V K2400_01" {
        n253 = local read "V K2400_01 array"() -> (w252:dbl[])
      }
      frame "V K2400_02" {
        n254 = local read "V K2400_02 array"() -> (w253:dbl[])
      }
      frame "I K2400_01" {
        n255 = local read "I K2400 01"() -> (w254:dbl[])
      }
      frame "I K2400_02" {
        n256 = local read "I K2400 02"() -> (w255:dbl[])
      }
      frame "DMM1" {
        n257 = local read "Voltage DMM1"() -> (w256:dbl[])
      }
      frame "DMM2" {
        n258 = local read "Voltage DMM2"() -> (w257:dbl[])
      }
      frame "B" {
        n259 = local read "B"() -> (w258:dbl[])
      }
      frame "R4probe" {
        n260 = local read "R4probe array"() -> (w259:dbl[])
      }
      frame "Formula1" {
        n261 = local read "Formula1Array"() -> (w260:dbl[])
      }
      frame "Formula2" {
        n262 = local read "Formula2Array"() -> (w261:dbl[])
      }
      frame "Formula3" {
        n263 = local read "Formula3Array"() -> (w262:dbl[])
      }
      frame "Formula4" {
        n264 = local read "Formula4Array"() -> (w263:dbl[])
      }
    }
    n265 = call "AxisLabel.vi"("Axis"="X-Axis 1") -> ("X Scale.Name Label.Text"=w38:string)
    n266 = call "AxisLabel.vi"("Axis"="Y-Axis 1") -> ("X Scale.Name Label.Text"=w37:string)
    n267 = property on="Fig 2" class="XYGraph (strict)"("XScale.NameLbl.Text"=w41) -> ()  [unwired: 2 in, 2 out]
    n268 = call "AxisLabel.vi"("Axis"="X-Axis 4") -> ("X Scale.Name Label.Text"=w24:string)
    n269 = call "AxisLabel.vi"("Axis"="Y-Axis 4") -> ("X Scale.Name Label.Text"=w25:string)
    n270 = Decimal String To Number(string="Fig3 Y scale 2") -> (number=w23:i32)  [unwired: 2 in, 1 out]
    n271 = call "AxisLabel.vi"("Axis"="X-Axis 3") -> ("X Scale.Name Label.Text"=w30:string)
    n272 = Decimal String To Number(string="Fig3 Y scale") -> (number=w28:i32)  [unwired: 2 in, 1 out]
    n273 = Decimal String To Number(string="Fig2 Y scale") -> (number=w34:i32)  [unwired: 2 in, 1 out]
    n274 = Decimal String To Number(string="Fig1 Y scale") -> (number=w32:i32)  [unwired: 2 in, 1 out]
    n275 = property on="Isd 4" class="XYGraph (strict)"("XScale.NameLbl.Text"=w24, "YScale.NameLbl.Text"=w25, "YScale.Mapping Mode"=w23) -> ()  [unwired: 2 in, 2 out]
    n276 = event shown="[1] \"Sensitivity Lockin1\", \"Sensitivity Lockin2\": Value Change" {
      selector: _ -> [_ _]
      dyn-events: _ -> [_ _]
      timeout: w40 -> [_ _]
      tunnel: w44 -> [w295 w296]
      tunnel: [w295 w296] -> w43
      event Timeout {
        n277 = event-data() -> ()  [unwired: 1 in, 2 out]
      }
      event "Sensitivity Lockin1", "Sensitivity Lockin2": Value Change {
        w297 = TRUE ("Change sensitivity ?")
        n278 = event-data() -> ()  [unwired: 1 in, 5 out]
        n279 = local read "Lockin1"() -> (w301:refnum<visa-resource-name>)
        n280 = local read "Lockin2"() -> (w300:refnum<visa-resource-name>)
        n281 = call "Sr830sens_giulia.vi"("Sr 830 sensitivity"="Sensitivity Lockin1", "Change sensitivity ?"=w297, "SR830"=w301) -> ()  [unwired: 1 out]
        n282 = call "Sr830sens_giulia.vi"("Sr 830 sensitivity"="Sensitivity Lockin2", "Change sensitivity ?"=w297, "SR830"=w300) -> ()  [unwired: 1 out]
      }
    }
    n283 = property on="Isd 3" class="XYGraph (strict)"("XScale.NameLbl.Text"=w30, "YScale.NameLbl.Text"=w29, "YScale.Mapping Mode"=w28) -> ()  [unwired: 2 in, 2 out]
    n284 = property on="Fig 2" class="XYGraph (strict)"("YScale.NameLbl.Text"=w42, "YScale.Mapping Mode"=w34) -> ()  [unwired: 2 in, 2 out]
    n285 = property on="Isd" class="XYGraph (strict)"("XScale.NameLbl.Text"=w38, "YScale.NameLbl.Text"=w37, "YScale.Mapping Mode"=w32) -> ()  [unwired: 2 in, 2 out]
    n286 = local read "stopMainLoop"() -> (w45:bool)
    n287 = Bundle("Formula4Array"=w18, "Formula4Array"=w16) -> (→"Isd 4":T7)  [unwired: 1 out]
    n288 = Bundle("Formula4Array"=w13, "Formula4Array"=w14) -> (→"Isd 3":T7)  [unwired: 1 out]
    n289 = Bundle("Formula4Array"=w8, "Formula4Array"=w9) -> (→"Fig 2":T7)  [unwired: 1 out]
    n290 = Bundle("Formula4Array"=w22, "Formula4Array"=w19) -> (→"Isd":T7)  [unwired: 1 out]
  }
  n291 = while {
    shift-right: [w329] -> _
    shift-left: "start" -> [w330]
    tunnel: w5 -> [w326]
    stop <- w325 stop-if-true
    n292 = case shown="\"measureOutParam\"" w330 {
      tunnel: ["measureSetInstruments" "measureSignal" "measureOutParam" "Calculate" "measureSetInstruments" "writeFile" ""] -> w329
      tunnel: [_ _ _ _ _ _ TRUE ("x")] -> w327
      tunnel: w326 -> [_ _ _ w558 _ _ _]
      tunnel: [_ _ _ _ w580 _ _] -> _
      tunnel: [_ _ _ _ _ w666 _] -> _
      tunnel: [_ _ _ _ _ w656 _] -> _
      tunnel: [_ _ _ _ _ w655 _] -> _
      tunnel: [_ _ _ _ _ w654 _] -> _
      frame "start", Default {
        w339 = "\t"
        w346 = "\t"
        w354 = "\t"
        w335 = "\t"
        w361 = "\t"
        w355 = "\t"
        w370 = "\t"
        # "Time\nT\nB\nWavelength\nDAC\nV K2400_01\nV K2400_02\nLockin V\nDMM1\nDMM2\nLK 1 X\nLK 1 Y\nLK2 X\nLK2 Y\nI K2400_01\nI K2400_02\nVsd\nVbgate\nVtopgate\nI2probe\nIleak bg\nIleak tg\nVxx\nVxy\nR2probe\nR4probe"
        n293 = Initialize Array(0) -> (→"Time" →"T" →"DAC 1 array" →"V K2400_01 array" →"V K2400_02 array" →"Lockin1 Y" →"Lockin1 X" →"Lockin2 Y" →"Lockin2 X" →"B" →"Voltage DMM1" →"Voltage DMM2" →"I K2400 02" →"I K2400 01" →"Wavelength array" →"Vbg array" →"Vtg array" →"Vsd array" →"Isd array" →"Vxx array" →"Vxy array" →"Ibg array" →"Itg array" →"R2probe array" →"R4probe array" →"Rxy Array" →"DAC 2 array":i32[])  [unwired: 1 out]
        n294 = Get Date/Time In Seconds() -> (seconds since 1Jan1904=w384:timestamp)
        n295 = Concatenate Strings("I 2probe [nA]" ("string"), w346, "Ileak bg [nA]" ("string"), w346, "Ileak tg [nA]" ("string"), w346) -> (w344:string)
        n296 = Get Date/Time String(date format (0)=1, seconds (now)=w384) -> (date string=w381:string, time string=w382:string)  [unwired: 1 out]
        n297 = Concatenate Strings("Vxx [V]" ("string"), w339, "Vxy [V]" ("string"), w339, "R2probe [kOhm]" ("string"), w339, "R4probe [kOhm]" ("string")) -> (w338:string)
        n298 = Concatenate Strings(w382, "\t", w381, "\r\n") -> (w377:string)
        n299 = Concatenate Strings("DMM1 [V]" ("string"), w361, "DMM2 [V]" ("string"), w361, "Lockin1 X [V]" ("string"), w361, "Lockin1 Y [V]" ("string"), w361, "Lockin2 X [V]" ("string"), w361, "Lockin2 Y [V]" ("string"), w361) -> (w357:string)
        n300 = Concatenate Strings("DAC 1 [V]" ("string"), w335, "DAC 2 [V]" ("string"), w335, "K2400_01 [V]" ("string"), w335, "K2400_02 [V]" ("string"), w335, "Lockin V [V]" ("string"), w335) -> (w358:string)
        n301 = Concatenate Strings("Time [s]", w370, "T [K]" ("chaîne"), w370, "B [T]" ("chaîne"), w370, "Wavelength [nm]" ("chaîne"), w370) -> (w376:string)
        n302 = Concatenate Strings("Vsd [V]" ("string"), w354, "Vbg [V]" ("string"), w354, "Vtg [V]" ("string"), w354) -> (w350:string)
        n303 = Concatenate Strings("I K2400_01 [A]" ("string"), w355, "I K2400_02 [A]" ("string"), w355) -> (w356:string)
        n304 = local read "File Name"() -> (w388:path)
        n305 = Concatenate Strings(w377, w376, w358, w357, w356, w350, w344, w338, "\r\n") -> (w378:string)
        n306 = Open/Create/Replace File(file path (use dialog)=w388, prompt="Enter data filename", operation (0:open)=5) -> (refnum out=w385:refnum<file>, error out=w374:errorcluster)  [unwired: 1 in, 3 out]
        n307 = Write to Text File(file (use dialog)=w385, text=w378, error in=w374) -> (refnum out=→"refnum out":refnum<file>, error out=w337:errorcluster)  [unwired: 2 out]
        n308 = case shown="No Error" w337 {
          frame No Error {
          }
          frame Error {
          }
        }
      }
      frame "measureSetInstruments" {
        w403 = errorcluster {"status"=FALSE, "code"=0, "source"=""} ("error in (no error)")
        w398 = 0.0
        n309 = local read "K2400_1"() -> (w421:bool)
        n310 = local read "K2400_2"() -> (w420:bool)
        n311 = local read "K2400 1"() -> (w413:refnum<visa-resource-name>)
        n312 = local read "K2400 2"() -> (w412:refnum<visa-resource-name>)
        n313 = local read "Lockin1 present"() -> (w410:bool)
        n314 = local read "Lockin1"() -> (w411:refnum<visa-resource-name>)
        n315 = case shown="True" w421 {
          tunnel: [w459 w464] -> w407
          tunnel: w398 -> [w459 _]
          tunnel: w413 -> [_ w463]
          tunnel: w403 -> [_ _]
          tunnel: [w459 w460] -> w402
          frame False {
          }
          frame True {
            n316 = call "K2400_write&read.vi"("Command"="READ?", "VISA Resource Name"=w463) -> ("error out"=w462:errorcluster, "Read"=w468:string)  [unwired: 1 in]
            n317 = case shown="No Error" w462 {
              frame No Error {
              }
              frame Error {
              }
            }
            n318 = Match Pattern(string=w468, regular expression=",") -> (before substring=w465:string, after substring=w461:string)  [unwired: 3 out]
            n319 = Fract/Exp String To Number(string=w465) -> (number=w464:dbl)  [unwired: 4 out]
            n320 = Fract/Exp String To Number(string=w461) -> (number=w460:dbl)  [unwired: 4 out]
          }
        }
        "I K2400_1 [A]" <- w402
        n321 = case shown="True" w420 {
          tunnel: [w448 w454] -> w405
          tunnel: w398 -> [w448 _]
          tunnel: w412 -> [_ w453]
          tunnel: w403 -> [_ w452]
          tunnel: [w448 w449] -> w401
          frame False {
          }
          frame True {
            n322 = call "K2400_write&read.vi"("error in (no error)"=w452, "Command"="READ?", "VISA Resource Name"=w453) -> ("error out"=w451:errorcluster, "Read"=w458:string)
            n323 = case shown="No Error" w451 {
              frame No Error {
              }
              frame Error {
              }
            }
            n324 = Match Pattern(string=w458, regular expression=",") -> (before substring=w455:string, after substring=w450:string)  [unwired: 3 out]
            n325 = Fract/Exp String To Number(string=w455) -> (number=w454:dbl)  [unwired: 4 out]
            n326 = Fract/Exp String To Number(string=w450) -> (number=w449:dbl)  [unwired: 4 out]
          }
        }
        "I K2400_2 [A]" <- w401
        n327 = global read "DACreadglobal.vi" "DAC read global (mV)"() -> (w392:dbl[])
        n328 = local read "DAC number 1"() -> (w409:u8)
        n329 = local read "DAC present"() -> (w395:bool)
        n330 = case shown="True" w410 {
          tunnel: [w430 w432] -> w406
          tunnel: w398 -> [w430 _]
          tunnel: w411 -> [_ w431]
          frame False {
          }
          frame True {
            n331 = VISA Write(VISA resource name=w431, write buffer="SLVL? " ("chaîne")) -> (VISA resource name out=w436:refnum<visa-resource-name>, error out=w435:errorcluster)  [unwired: 1 in, 1 out]
            n332 = VISA Read(VISA resource name=w436, byte count=u32 1024, error in (no error)=w435) -> (read buffer=w433:string)  [unwired: 3 out]
            n333 = Fract/Exp String To Number(string=w433) -> (number=w432:dbl)  [unwired: 4 out]
          }
        }
        n334 = local read "DAC"() -> (w399:refnum<visa-resource-name>)
        n335 = case shown="True" w395 {
          selector: w395 -> [w439 w445]
          tunnel: [w440 w446] -> w408
          tunnel: w398 -> [w440 _]
          tunnel: w399 -> [_ _]
          tunnel: w409 -> [_ w444]
          tunnel: [w439 w445] -> w393
          tunnel: w392 -> [w438 w441]
          tunnel: [w438 w441] -> w391
          frame False {
          }
          frame True {
            n336 = Decrement(x=w444) -> (x-1=w443:u8)
            n337 = Index Array(array=w441, index=w443) -> (element=w442:dbl)
            n338 = Divide(x=w442, y=1000.0) -> (x/y=w446:dbl)
          }
        }
        n339 = local read "DAC number 2"() -> (w400:u8)
        n340 = local read "DAC 1 array"() -> (w419:dbl[])
        n341 = local read "V K2400_01 array"() -> (w416:dbl[])
        n342 = local read "V K2400_02 array"() -> (w417:dbl[])
        n343 = local write "Lockin1 Ampl [V]"(w406) -> ()
        n344 = case shown="True" w393 {
          tunnel: [w423 w428] -> w394
          tunnel: w398 -> [w423 _]
          tunnel: w399 -> [_ _]
          tunnel: w400 -> [_ w425]
          tunnel: w391 -> [_ w426]
          frame False {
          }
          frame True {
            n345 = Decrement(x=w425) -> (x-1=w427:u8)
            n346 = Index Array(array=w426, index=w427) -> (element=w424:dbl)
            n347 = Divide(x=w424, y=1000.0) -> (x/y=w428:dbl)
          }
        }
        n348 = local write "DAC 1 V [V]"(w408) -> ()
        n349 = Build Array (concatenate)(w419, w408) -> (w418:dbl[])
        n350 = local write "K2400 1 [V]"(w407) -> ()
        n351 = local write "K2400 2 [V]"(w405) -> ()
        n352 = local write "DAC 1 array"(w418) -> ()
        n353 = Build Array (concatenate)(w416, w407) -> (w414:dbl[])
        n354 = Build Array (concatenate)(w417, w405) -> (w415:dbl[])
        n355 = local write "V K2400_01 array"(w414) -> ()
        n356 = local write "V K2400_02 array"(w415) -> ()
        n357 = local read "DAC 2 array"() -> (w397:dbl[])
        n358 = local write "DAC 2 V [V]"(w394) -> ()
        n359 = Bundle(w408, w407, w405, w406, w394) -> (→"SetIntr Cluster":cluster{dbl, dbl, dbl, dbl, dbl})  [unwired: 1 in]
        n360 = Build Array (concatenate)(w397, w394) -> (w396:dbl[])
        n361 = local write "DAC 2 array"(w396) -> ()
      }
      frame "measureSignal" {
        w500 = 0.0
        n362 = local read "K2400_1"() -> (w511:bool)
        n363 = local read "K2400 1"() -> (w512:refnum<visa-resource-name>)
        n364 = local read "DMM1"() -> (w507:bool)
        n365 = local read "DMM1"() -> (w508:refnum<visa-resource-name>)
        n366 = local read "Lockin1 present"() -> (w509:bool)
        n367 = local read "Lockin1"() -> (w510:refnum<visa-resource-name>)
        n368 = case shown="True" w507 {
          tunnel: w508 -> [_ w529]
          tunnel: [w525 w528] -> w473
          tunnel: w500 -> [w525 w527]
          tunnel: [w525 w527] -> w476
          frame False {
          }
          frame True {
            n369 = call "AGILENT34401a_read.vi"("VISA Resource Name in"=w529) -> ("Voltage output"=w528:dbl, "error out"=w526:errorcluster)  [unwired: 1 out]
            n370 = case shown="No Error" w526 {
              frame No Error {
              }
              frame Error {
              }
            }
          }
        }
        "V DMM1 [V]" <- w473
        n371 = case shown="False" w511 {
          tunnel: [w531 w532] -> w471
          tunnel: w512 -> [_ _]
          tunnel: w500 -> [w531 _]
          tunnel: "READ?" -> [w530 w533]
          tunnel: [w530 w533] -> w478
          frame False {
          }
          frame True {
            n372 = local read "I K2400_1 [A]"() -> (w532:dbl)
          }
        }
        n373 = case shown="True" w509 {
          tunnel: w510 -> [_ w540]
          tunnel: [w534 w539] -> w475
          tunnel: [w534 w538] -> w488
          tunnel: w500 -> [w534 w536]
          tunnel: [w535 w537] -> w480
          tunnel: "1,4" ("Variable") -> [w535 w537]
          tunnel: [w534 w536] -> w477
          frame False {
          }
          frame True {
            n374 = call "Lockin_SR830_readXY.vi"("Variable"=w537, "VISA Resource Name"=w540) -> ("Output Y"=w538:dbl, "Output X"=w539:dbl)
          }
        }
        "Lockin1 X [V]" <- w475
        "Lockin1 Y [V]" <- w488
        n375 = local read "I K2400 01"() -> (w499:dbl[])
        n376 = local read "K2400_2"() -> (w501:bool)
        n377 = local read "K2400 2"() -> (w502:refnum<visa-resource-name>)
        n378 = local read "Lockin2 present"() -> (w503:bool)
        n379 = local read "Lockin1 Y"() -> (w489:dbl[])
        n380 = local read "Lockin1 X"() -> (w492:dbl[])
        n381 = local read "Lockin2"() -> (w504:refnum<visa-resource-name>)
        n382 = case shown="False" w501 {
          tunnel: [w514 w515] -> w469
          tunnel: w502 -> [_ _]
          tunnel: w500 -> [w514 _]
          tunnel: w478 -> [_ _]
          frame False {
          }
          frame True {
            n383 = local read "I K2400_2 [A]"() -> (w515:dbl)
          }
        }
        n384 = Build Array (concatenate)(w499, w471) -> (w498:dbl[])
        n385 = local read "Voltage DMM1"() -> (w484:dbl[])
        n386 = local read "DMM2"() -> (w506:bool)
        n387 = local read "DMM2"() -> (w505:refnum<visa-resource-name>)
        n388 = case shown="True" w503 {
          tunnel: w504 -> [_ w520]
          tunnel: [w516 w519] -> w474
          tunnel: [w516 w518] -> w494
          tunnel: w477 -> [w516 _]
          tunnel: w480 -> [_ w517]
          frame False {
          }
          frame True {
            n389 = call "Lockin_SR830_readXY.vi"("Variable"=w517, "VISA Resource Name"=w520) -> ("Output Y"=w518:dbl, "Output X"=w519:dbl)
          }
        }
        "Lockin2 X [V]" <- w474
        "Lockin2 Y [V]" <- w494
        n390 = local write "I K2400 01"(w498) -> ()
        n391 = Build Array (concatenate)(w489, w488) -> (w490:dbl[])
        n392 = Build Array (concatenate)(w492, w475) -> (w491:dbl[])
        n393 = case shown="True" w506 {
          tunnel: w505 -> [_ w524]
          tunnel: [w521 w523] -> w472
          tunnel: w476 -> [w521 _]
          frame False {
          }
          frame True {
            n394 = call "AGILENT34401a_read.vi"("VISA Resource Name in"=w524) -> ("Voltage output"=w523:dbl, "error out"=w522:errorcluster)  [unwired: 1 out]
            n395 = case shown="No Error" w522 {
              frame No Error {
              }
              frame Error {
              }
            }
          }
        }
        "V DMM2 [V]" <- w472
        n396 = local write "Lockin1 Y"(w490) -> ()
        n397 = local write "Lockin1 X"(w491) -> ()
        n398 = Build Array (concatenate)(w484, w473) -> (w482:dbl[])
        n399 = local write "Voltage DMM1"(w482) -> ()
        n400 = local read "I K2400 02"() -> (w486:dbl[])
        n401 = local read "Lockin2 Y"() -> (w495:dbl[])
        n402 = local read "Lockin2 X"() -> (w497:dbl[])
        n403 = Build Array (concatenate)(w486, w469) -> (w487:dbl[])
        n404 = local write "I K2400 02"(w487) -> ()
        n405 = Build Array (concatenate)(w495, w494) -> (w493:dbl[])
        n406 = Build Array (concatenate)(w497, w474) -> (w496:dbl[])
        n407 = local write "Lockin2 Y"(w493) -> ()
        n408 = local write "Lockin2 X"(w496) -> ()
        n409 = local read "Voltage DMM2"() -> (w485:dbl[])
        n410 = Bundle("Output X"=w475, "Output X"=w474, "Voltage output"=w473, "Voltage output"=w472, "I K2400_1 [A]"=w471, "I K2400_2 [A]"=w469) -> (→"signal cluster":T8)  [unwired: 1 in]
        n411 = Build Array (concatenate)(w485, w472) -> (w483:dbl[])
        n412 = local write "Voltage DMM2"(w483) -> ()
      }
      frame "measureOutParam" {
        w545 = 0.0
        n413 = Tick Count (ms)() -> (millisecond timer value=w561:u32)
        n414 = local read "Wvlen query"() -> (w544:bool)
        n415 = local read "Bfield query"() -> (w556:bool)
        n416 = Subtract(x=w561, y=w558) -> (x-y=w559:u32)
        n417 = local read "Tcontrol"() -> (w557:string)
        n418 = case shown="True" w556 {
          tunnel: [w567 w568] -> w550
          tunnel: w545 -> [w567 _]
          frame False {
          }
          frame True {
            n419 = call "TeslReadField.vi"() -> ("Effective field"=w569:dbl[unit])  [unwired: 6 in, 1 out]
            n420 = node(w569) -> (w568:dbl)
          }
        }
        "B [T]" <- w550
        n421 = case shown="True" w544 {
          tunnel: w545 -> [w563 _]
          tunnel: [w563 w565] -> w542
          tunnel: [_ w564] -> _
          frame False {
          }
          frame True {
            n422 = global read "perHandlemonochromator.vi" "peHandle"() -> (w566:u32)
            n423 = call "PE Get Wavelength.vi"("peHandle"=w566) -> ("error out"=w564:errorcluster, "wavelength"=w565:dbl)  [unwired: 8 in, 1 out]
          }
        }
        "Wavelength [nm]" <- w542
        n424 = local read "TIC"() -> (w549:refnum<visa-resource-name>)
        n425 = Quotient & Remainder(x=w559, y=u32 1000) -> (floor(x/y)=w546:u32)  [unwired: 1 out]
        "Time [s]" <- w546
        n426 = case shown="\"GlobalVar\"" w557 {
          tunnel: [0.0 w572 w576 w578] -> w553
          tunnel: w549 -> [_ w571 _ _]
          frame "OFF", Default {
          }
          frame "TIC (OeLab)" {
            n427 = call "TIC_rw.vi"("write buffer"="in1.value?", "TIC 500"=w571) -> ("read buffer"=w574:string)  [unwired: 1 in, 2 out]
            n428 = Scan Value(string=w574, format string="%.3f") -> (value=w572:dbl)  [unwired: 1 in, 1 out]
          }
          frame "ITC" {
            n429 = local read "ITC signal"() -> (w577:T1)
            n430 = call "ITCGetReading.vi"("Signal"=w577) -> ("Reading"=w576:dbl)  [unwired: 6 in]
          }
          frame "GlobalVar" {
            n431 = global read "Tglobalvar.vi" "Tglobalvar"() -> (w578:dbl)
          }
        }
        "T [K]" <- w553
        n432 = local read "Time"() -> (w547:dbl[])
        n433 = Build Array (concatenate)(w547, w546) -> (w548:dbl[])
        n434 = local write "Time"(w548) -> ()
        n435 = local read "Wavelength array"() -> (w543:dbl[])
        n436 = Build Array (concatenate)(w543, w542) -> (w541:dbl[])
        n437 = local read "B"() -> (w552:dbl[])
        n438 = local write "Wavelength array"(w541) -> ()
        n439 = Build Array (concatenate)(w552, w550) -> (w551:dbl[])
        n440 = local write "B"(w551) -> ()
        n441 = local read "T"() -> (w554:dbl[])
        n442 = Build Array (concatenate)(w554, w553) -> (w555:dbl[])
        n443 = local write "T"(w555) -> ()
      }
      frame "writeFile" {
        n444 = local read "SaveDataQuery"() -> (w579:bool)
        n445 = case shown="True" w579 {
          frame False {
          }
          frame True {
            w590 = "\t"
            w601 = "\t"
            w608 = "\t"
            w588 = "\t"
            w625 = "\t"
            w585 = "\t"
            w616 = "\t"
            # "Time\nT\nB\nWavelength\nDAC\nV K2400_01\nV K2400_02\nLockin V\nDMM1\nDMM2\nLK 1 X\nLK 1 Y\nLK2 X\nLK2 Y\nI K2400_01\nI K2400_02\nVsd\nVbgate\nVtopgate\nI2probe\nIleak bg\nIleak tg\nVxx\nVxy\nR2probe\nR4probe"
            # "I K2400_01\nI K2400_02"
            # "DMM1\nDMM2\nLK 1 X\nLK 1 Y\nLK2 X\nLK2 Y"
            # "DAC\nV K2400_01\nV K2400_02\nLockin V"
            # "Time\nT\nB\nWavelength"
            # "Time\nT\nB\nDAC\nV K2400_01\nV K2400_02\nLockin V\nDMM1\nDMM2\nLK 1 X\nLK 1 Y\nLK2 X\nLK2 Y\nI K2400_01\nI K2400_02"
            n446 = local read "Lockin1 Ampl [V]"() -> (w641:dbl)
            n447 = local read "Wavelength [nm]"() -> (w618:dbl)
            n448 = local read "R 2probe [kOhm]"() -> (w596:dbl)
            n449 = local read "R 4probe [kOhm]"() -> (w595:dbl)
            n450 = local read "V_backgate [V]"() -> (w612:dbl)
            n451 = local read "I Leak BG [nA]"() -> (w604:dbl)
            n452 = local read "I Leak TG[nA]"() -> (w605:dbl)
            n453 = local read "V_topgate [V]"() -> (w611:dbl)
            n454 = local read "I 2probe [nA]"() -> (w606:dbl)
            n455 = local read "Lockin1 X [V]"() -> (w635:dbl)
            n456 = local read "Lockin1 Y [V]"() -> (w634:dbl)
            n457 = local read "Lockin2 X [V]"() -> (w633:dbl)
            n458 = local read "Lockin2 Y [V]"() -> (w632:dbl)
            n459 = local read "I K2400_1 [A]"() -> (w624:dbl)
            n460 = local read "V DMM1 [V]"() -> (w637:dbl)
            n461 = local read "V DMM2 [V]"() -> (w636:dbl)
            n462 = local read "DAC 1 V [V]"() -> (w587:dbl)
            n463 = local read "DAC 2 V [V]"() -> (w584:dbl)
            n464 = local read "K2400 1 [V]"() -> (w645:dbl)
            n465 = local read "K2400 2 [V]"() -> (w643:dbl)
            n466 = local read "Time [s]"() -> (w652:dbl)
            n467 = local read "T [K]"() -> (w650:dbl)
            n468 = local read "Vsd [V]"() -> (w614:dbl)
            n469 = local read "Vxx [V]"() -> (w598:dbl)
            n470 = local read "Vxy [V]"() -> (w597:dbl)
            n471 = local read "B [T]"() -> (w648:dbl)
            n472 = Number To Exponential String(number=w587) -> (E-format string=w586:string)  [unwired: 3 in]
            n473 = Number To Exponential String(number=w584) -> (E-format string=w583:string)  [unwired: 3 in]
            n474 = Number To Exponential String(number=w645) -> (E-format string=w644:string)  [unwired: 3 in]
            n475 = Number To Exponential String(number=w643) -> (E-format string=w642:string)  [unwired: 3 in]
            n476 = Number To Exponential String(number=w641) -> (E-format string=w640:string)  [unwired: 3 in]
            n477 = Number To Exponential String(number=w606) -> (E-format string=w600:string)  [unwired: 3 in]
            n478 = Number To Exponential String(number=w604) -> (E-format string=w602:string)  [unwired: 3 in]
            n479 = Number To Exponential String(number=w605) -> (E-format string=w603:string)  [unwired: 3 in]
            n480 = Number To Exponential String(number=w652) -> (E-format string=w651:string)  [unwired: 3 in]
            n481 = Number To Exponential String(number=w650) -> (E-format string=w649:string)  [unwired: 3 in]
            n482 = Number To Exponential String(number=w648) -> (E-format string=w647:string)  [unwired: 3 in]
            n483 = Number To Exponential String(number=w618) -> (E-format string=w617:string)  [unwired: 3 in]
            n484 = Number To Exponential String(number=w637) -> (E-format string=w631:string)  [unwired: 3 in]
            n485 = Number To Exponential String(number=w636) -> (E-format string=w630:string)  [unwired: 3 in]
            n486 = Number To Exponential String(number=w635) -> (E-format string=w629:string)  [unwired: 3 in]
            n487 = Number To Exponential String(number=w634) -> (E-format string=w628:string)  [unwired: 3 in]
            n488 = Number To Exponential String(number=w633) -> (E-format string=w627:string)  [unwired: 3 in]
            n489 = Number To Exponential String(number=w632) -> (E-format string=w626:string)  [unwired: 3 in]
            n490 = Number To Exponential String(number=w614) -> (E-format string=w613:string)  [unwired: 3 in]
            n491 = Number To Exponential String(number=w612) -> (E-format string=w610:string)  [unwired: 3 in]
            n492 = Number To Exponential String(number=w611) -> (E-format string=w609:string)  [unwired: 3 in]
            n493 = Number To Exponential String(number=w598) -> (E-format string=w594:string)  [unwired: 3 in]
            n494 = Number To Exponential String(number=w597) -> (E-format string=w593:string)  [unwired: 3 in]
            n495 = Number To Exponential String(number=w596) -> (E-format string=w592:string)  [unwired: 3 in]
            n496 = Number To Exponential String(number=w595) -> (E-format string=w591:string)  [unwired: 3 in]
            n497 = local read "I K2400_2 [A]"() -> (w623:dbl)
            n498 = Concatenate Strings(w613, w608, w610, w608, w609, w608) -> (w607:string)
            n499 = Concatenate Strings(w586, w585, w583, w585, w644, w585, w642, w585, w640, w585) -> (w639:string)
            n500 = Concatenate Strings(w600, w601, w602, w601, w603, w601) -> (w599:string)
            n501 = Concatenate Strings(w631, w625, w630, w625, w629, w625, w628, w625, w627, w625, w626, w625) -> (w638:string)
            n502 = Concatenate Strings(w651, w616, w649, w616, w647, w616, w617, w616) -> (w646:string)
            n503 = Concatenate Strings(w594, w590, w593, w590, w592, w590, w591) -> (w589:string)
            n504 = Number To Exponential String(number=w624) -> (E-format string=w622:string)  [unwired: 3 in]
            n505 = Number To Exponential String(number=w623) -> (E-format string=w621:string)  [unwired: 3 in]
            n506 = Concatenate Strings(w622, w588, w621, w588) -> (w620:string)
            n507 = local read "refnum out"() -> (w653:refnum<file>)
            n508 = Concatenate Strings(w646, w639, w638, w620, w607, w599, w589, "\r\n") -> (w619:string)
            n509 = Write to Text File(file (use dialog)=w653, text=w619) -> ()  [unwired: 1 in, 4 out]
          }
        }
        n510 = local read "Refresh Rate [ms]"() -> (w581:i32)
        n511 = call "wait.vi"("wait time (ms)"=w581) -> ("error in (no error) 2"=w580:errorcluster)  [unwired: 1 in]
      }
      frame "Calculate" {
        w660 = string[] ["Temperature", "B", "Wavelength", "Vsd", "Isd", "Vbg", "Vtg", "Ibg", "Itg", "Vxx", "Vxy", "R2probe", "R4probe", "Rxy"] ("Axis select")
        # "lockin1 X\nLockin2 X\nDMM1\nDMM2\nI K2400 01\nI K2400 02"
        # "DAC 1\nK2400 1\nK2400 2\nLockin\nDAC 2"
        n512 = local read "Gain Cluster 2"() -> (w699:T3)
        n513 = local read "SetIntr Cluster"() -> (w752:cluster{dbl, dbl, dbl, dbl, dbl})
        n514 = local read "signal cluster"() -> (w753:T5)
        n515 = Unbundle By Name(w699) -> ("Vsd"=w700:string, "I 2probe 2"=w701:string, "Vxx"=w702:string, "Vxy"=w703:string, "V BG"=w704:string, "I leak BG"=w705:string, "V TG"=w706:string, "I leak TG"=w707:string)
        n516 = case shown="\"DAC 2 V\"" w704 {
          tunnel: w752 -> [w783 _ _ w789 w791 _ _ w797 w799 _ _]
          tunnel: w753 -> [_ w785 w787 _ _ w793 w795 _ _ w801 w803]
          tunnel: [w782 w784 w786 w788 w790 w792 w794 w796 w798 w800 w802] -> w744
          frame "LockinAmpl", Default {
            n517 = Unbundle(w783) -> (w782:dbl)  [unwired: 4 out]
          }
          frame "Lockin1 X" {
            n518 = Unbundle(w785) -> ("Output X"=w784:dbl)  [unwired: 5 out]
          }
          frame "Lockin2 X" {
            n519 = Unbundle(w787) -> ("Output X"=w786:dbl)  [unwired: 5 out]
          }
          frame "V K2400_01" {
            n520 = Unbundle(w789) -> (w788:dbl)  [unwired: 4 out]
          }
          frame "V K2400_02" {
            n521 = Unbundle(w791) -> (w790:dbl)  [unwired: 4 out]
          }
          frame "DMM1" {
            n522 = Unbundle(w793) -> ("Voltage output"=w792:dbl)  [unwired: 5 out]
          }
          frame "DMM2" {
            # "BG"
            n523 = Unbundle(w795) -> ("Voltage output"=w794:dbl)  [unwired: 5 out]
          }
          frame "DAC 1 V" {
            n524 = Unbundle(w797) -> (w796:dbl)  [unwired: 4 out]
          }
          frame "DAC 2 V" {
            n525 = Unbundle(w799) -> (w798:dbl)  [unwired: 4 out]
          }
          frame "I K2400_01" {
            n526 = Unbundle(w801) -> (w800:dbl)  [unwired: 5 out]
          }
          frame "K2400_02" {
            n527 = Unbundle(w803) -> (w802:dbl)  [unwired: 5 out]
          }
        }
        n528 = case shown="\"DAC 2 V\"" w706 {
          tunnel: w752 -> [w761 _ _ w767 w769 _ _ w775 w777 _ _]
          tunnel: w753 -> [_ w763 w765 _ _ w771 w773 _ _ w779 w781]
          tunnel: [w760 w762 w764 w766 w768 w770 w772 w774 w776 w778 w780] -> w742
          frame "LockinAmpl", Default {
            n529 = Unbundle(w761) -> (w760:dbl)  [unwired: 4 out]
          }
          frame "Lockin1 X" {
            n530 = Unbundle(w763) -> ("Output X"=w762:dbl)  [unwired: 5 out]
          }
          frame "Lockin2 X" {
            n531 = Unbundle(w765) -> ("Output X"=w764:dbl)  [unwired: 5 out]
          }
          frame "V K2400_01" {
            n532 = Unbundle(w767) -> (w766:dbl)  [unwired: 4 out]
          }
          frame "V K2400_02" {
            n533 = Unbundle(w769) -> (w768:dbl)  [unwired: 4 out]
          }
          frame "DMM1" {
            n534 = Unbundle(w771) -> ("Voltage output"=w770:dbl)  [unwired: 5 out]
          }
          frame "DMM2" {
            # "TG"
            n535 = Unbundle(w773) -> ("Voltage output"=w772:dbl)  [unwired: 5 out]
          }
          frame "DAC 1 V" {
            n536 = Unbundle(w775) -> (w774:dbl)  [unwired: 4 out]
          }
          frame "DAC 2 V" {
            n537 = Unbundle(w777) -> (w776:dbl)  [unwired: 4 out]
          }
          frame "I K2400_01" {
            n538 = Unbundle(w779) -> (w778:dbl)  [unwired: 5 out]
          }
          frame "K2400_02" {
            n539 = Unbundle(w781) -> (w780:dbl)  [unwired: 5 out]
          }
        }
        n540 = case shown="\"DAC 2 V\"" w705 {
          tunnel: w752 -> [w871 _ _ w877 w879 _ _ w885 w887 _ _]
          tunnel: w753 -> [_ w873 w875 _ _ w881 w882 _ _ w889 w891]
          tunnel: [w870 w872 w874 w876 w878 w880 w883 w884 w886 w888 w890] -> w754
          frame "LockinAmpl", Default {
            n541 = Unbundle(w871) -> (w870:dbl)  [unwired: 4 out]
          }
          frame "Lockin1 X" {
            n542 = Unbundle(w873) -> ("Output X"=w872:dbl)  [unwired: 5 out]
          }
          frame "Lockin2 X" {
            n543 = Unbundle(w875) -> ("Output X"=w874:dbl)  [unwired: 5 out]
          }
          frame "V K2400_01" {
            n544 = Unbundle(w877) -> (w876:dbl)  [unwired: 4 out]
          }
          frame "V K2400_02" {
            n545 = Unbundle(w879) -> (w878:dbl)  [unwired: 4 out]
          }
          frame "DMM1" {
            n546 = Unbundle(w881) -> ("Voltage output"=w880:dbl)  [unwired: 5 out]
          }
          frame "DMM2" {
            # "leak BG"
            n547 = Unbundle(w882) -> ("Voltage output"=w883:dbl)  [unwired: 5 out]
          }
          frame "DAC 1 V" {
            n548 = Unbundle(w885) -> (w884:dbl)  [unwired: 4 out]
          }
          frame "DAC 2 V" {
            n549 = Unbundle(w887) -> (w886:dbl)  [unwired: 4 out]
          }
          frame "I K2400_01" {
            n550 = Unbundle(w889) -> (w888:dbl)  [unwired: 5 out]
          }
          frame "K2400_02" {
            n551 = Unbundle(w891) -> (w890:dbl)  [unwired: 5 out]
          }
        }
        n552 = case shown="\"DAC 2 V\"" w707 {
          tunnel: w752 -> [w849 _ _ w855 w857 _ _ w863 w865 _ _]
          tunnel: w753 -> [_ w851 w853 _ _ w859 w861 _ _ w867 w869]
          tunnel: [w848 w850 w852 w854 w856 w858 w860 w862 w864 w866 w868] -> w755
          frame "LockinAmpl", Default {
            n553 = Unbundle(w849) -> (w848:dbl)  [unwired: 4 out]
          }
          frame "Lockin1 X" {
            n554 = Unbundle(w851) -> ("Output X"=w850:dbl)  [unwired: 5 out]
          }
          frame "Lockin2 X" {
            n555 = Unbundle(w853) -> ("Output X"=w852:dbl)  [unwired: 5 out]
          }
          frame "V K2400_01" {
            n556 = Unbundle(w855) -> (w854:dbl)  [unwired: 4 out]
          }
          frame "V K2400_02" {
            n557 = Unbundle(w857) -> (w856:dbl)  [unwired: 4 out]
          }
          frame "DMM1" {
            n558 = Unbundle(w859) -> ("Voltage output"=w858:dbl)  [unwired: 5 out]
          }
          frame "DMM2" {
            # "leak TG"
            n559 = Unbundle(w861) -> ("Voltage output"=w860:dbl)  [unwired: 5 out]
          }
          frame "DAC 1 V" {
            n560 = Unbundle(w863) -> (w862:dbl)  [unwired: 4 out]
          }
          frame "DAC 2 V" {
            n561 = Unbundle(w865) -> (w864:dbl)  [unwired: 4 out]
          }
          frame "I K2400_01" {
            n562 = Unbundle(w867) -> (w866:dbl)  [unwired: 5 out]
          }
          frame "K2400_02" {
            n563 = Unbundle(w869) -> (w868:dbl)  [unwired: 5 out]
          }
        }
        n564 = case shown="\"DAC 2 V\"" w702 {
          tunnel: w752 -> [w827 _ _ w833 w835 _ _ w841 w843 _ _]
          tunnel: w753 -> [_ w829 w831 _ _ w837 w839 _ _ w845 w847]
          tunnel: [w826 w828 w830 w832 w834 w836 w838 w840 w842 w844 w846] -> w748
          frame "LockinAmpl", Default {
            n565 = Unbundle(w827) -> (w826:dbl)  [unwired: 4 out]
          }
          frame "Lockin1 X" {
            n566 = Unbundle(w829) -> ("Output X"=w828:dbl)  [unwired: 5 out]
          }
          frame "Lockin2 X" {
            n567 = Unbundle(w831) -> ("Output X"=w830:dbl)  [unwired: 5 out]
          }
          frame "V K2400_01" {
            n568 = Unbundle(w833) -> (w832:dbl)  [unwired: 4 out]
          }
          frame "V K2400_02" {
            n569 = Unbundle(w835) -> (w834:dbl)  [unwired: 4 out]
          }
          frame "DMM1" {
            n570 = Unbundle(w837) -> ("Voltage output"=w836:dbl)  [unwired: 5 out]
          }
          frame "DMM2" {
            # "Vxx"
            n571 = Unbundle(w839) -> ("Voltage output"=w838:dbl)  [unwired: 5 out]
          }
          frame "DAC 1 V" {
            n572 = Unbundle(w841) -> (w840:dbl)  [unwired: 4 out]
          }
          frame "DAC 2 V" {
            n573 = Unbundle(w843) -> (w842:dbl)  [unwired: 4 out]
          }
          frame "I K2400_01" {
            n574 = Unbundle(w845) -> (w844:dbl)  [unwired: 5 out]
          }
          frame "K2400_02" {
            n575 = Unbundle(w847) -> (w846:dbl)  [unwired: 5 out]
          }
        }
        n576 = case shown="\"DAC 2 V\"" w703 {
          tunnel: w752 -> [w805 _ _ w811 w813 _ _ w819 w821 _ _]
          tunnel: w753 -> [_ w807 w809 _ _ w815 w817 _ _ w823 w825]
          tunnel: [w804 w806 w808 w810 w812 w814 w816 w818 w820 w822 w824] -> w745
          frame "LockinAmpl", Default {
            n577 = Unbundle(w805) -> (w804:dbl)  [unwired: 4 out]
          }
          frame "Lockin1 X" {
            n578 = Unbundle(w807) -> ("Output X"=w806:dbl)  [unwired: 5 out]
          }
          frame "Lockin2 X" {
            n579 = Unbundle(w809) -> ("Output X"=w808:dbl)  [unwired: 5 out]
          }
          frame "V K2400_01" {
            n580 = Unbundle(w811) -> (w810:dbl)  [unwired: 4 out]
          }
          frame "V K2400_02" {
            n581 = Unbundle(w813) -> (w812:dbl)  [unwired: 4 out]
          }
          frame "DMM1" {
            n582 = Unbundle(w815) -> ("Voltage output"=w814:dbl)  [unwired: 5 out]
          }
          frame "DMM2" {
            # "Vxy"
            n583 = Unbundle(w817) -> ("Voltage output"=w816:dbl)  [unwired: 5 out]
          }
          frame "DAC 1 V" {
            n584 = Unbundle(w819) -> (w818:dbl)  [unwired: 4 out]
          }
          frame "DAC 2 V" {
            n585 = Unbundle(w821) -> (w820:dbl)  [unwired: 4 out]
          }
          frame "I K2400_01" {
            n586 = Unbundle(w823) -> (w822:dbl)  [unwired: 5 out]
          }
          frame "K2400_02" {
            n587 = Unbundle(w825) -> (w824:dbl)  [unwired: 5 out]
          }
        }
        n588 = case shown="\"DAC 2 V\"" w701 {
          tunnel: w752 -> [w893 _ _ w899 w901 _ _ w907 w909 _ _]
          tunnel: w753 -> [_ w895 w897 _ _ w903 w905 _ _ w911 w913]
          tunnel: [w892 w894 w896 w898 w900 w902 w904 w906 w908 w910 w912] -> w757
          frame "LockinAmpl", Default {
            n589 = Unbundle(w893) -> (w892:dbl)  [unwired: 4 out]
          }
          frame "Lockin1 X" {
            n590 = Unbundle(w895) -> ("Output X"=w894:dbl)  [unwired: 5 out]
          }
          frame "Lockin2 X" {
            n591 = Unbundle(w897) -> ("Output X"=w896:dbl)  [unwired: 5 out]
          }
          frame "V K2400_01" {
            n592 = Unbundle(w899) -> (w898:dbl)  [unwired: 4 out]
          }
          frame "V K2400_02" {
            n593 = Unbundle(w901) -> (w900:dbl)  [unwired: 4 out]
          }
          frame "DMM1" {
            n594 = Unbundle(w903) -> ("Voltage output"=w902:dbl)  [unwired: 5 out]
          }
          frame "DMM2" {
            # "I 2probe"
            n595 = Unbundle(w905) -> ("Voltage output"=w904:dbl)  [unwired: 5 out]
          }
          frame "DAC 1 V" {
            n596 = Unbundle(w907) -> (w906:dbl)  [unwired: 4 out]
          }
          frame "DAC 2 V" {
            n597 = Unbundle(w909) -> (w908:dbl)  [unwired: 4 out]
          }
          frame "I K2400_01" {
            n598 = Unbundle(w911) -> (w910:dbl)  [unwired: 5 out]
          }
          frame "K2400_02" {
            n599 = Unbundle(w913) -> (w912:dbl)  [unwired: 5 out]
          }
        }
        n600 = case shown="\"DAC 2 V\"" w700 {
          tunnel: w752 -> [w915 w918 _ w923 w925 _ _ w931 w933 _ _]
          tunnel: w753 -> [w916 w919 w921 _ _ w927 w929 _ _ w935 w937]
          tunnel: [w914 w917 w920 w922 w924 w926 w928 w930 w932 w934 w936] -> w759
          frame "LockinAmpl", Default {
            n601 = Unbundle(w916) -> ()  [unwired: 6 out]
            n602 = Unbundle(w915) -> (w914:dbl)  [unwired: 4 out]
          }
          frame "Lockin1 X" {
            n603 = Unbundle(w918) -> ()  [unwired: 5 out]
            n604 = Unbundle(w919) -> ("Output X"=w917:dbl)  [unwired: 5 out]
          }
          frame "Lockin2 X" {
            n605 = Unbundle(w921) -> ("Output X"=w920:dbl)  [unwired: 5 out]
          }
          frame "V K2400_01" {
            # "V sd"
            n606 = Unbundle(w923) -> (w922:dbl)  [unwired: 4 out]
          }
          frame "V K2400_02" {
            n607 = Unbundle(w925) -> (w924:dbl)  [unwired: 4 out]
          }
          frame "DMM1" {
            n608 = Unbundle(w927) -> ("Voltage output"=w926:dbl)  [unwired: 5 out]
          }
          frame "DMM2" {
            n609 = Unbundle(w929) -> ("Voltage output"=w928:dbl)  [unwired: 5 out]
          }
          frame "DAC 1 V" {
            n610 = Unbundle(w931) -> (w930:dbl)  [unwired: 4 out]
          }
          frame "DAC 2 V" {
            n611 = Unbundle(w933) -> (w932:dbl)  [unwired: 4 out]
          }
          frame "I K2400_01" {
            n612 = Unbundle(w935) -> (w934:dbl)  [unwired: 5 out]
          }
          frame "K2400_02" {
            n613 = Unbundle(w937) -> (w936:dbl)  [unwired: 5 out]
          }
        }
        n614 = Unbundle By Name(w699) -> ("I Gain 1"=w719:dbl, "V Gain 1"=w723:dbl, "conversion factor BG"=w721:dbl, "Vin / Vout 1"=w722:dbl, "V Gain 2"=w713:dbl, "Vin / Vout 2"=w712:dbl, "V Gain 3"=w711:dbl, "Vin / Vout 3"=w710:dbl, "I Gain 2"=w715:dbl, "I Gain 3"=w718:dbl, "conversion factor TG"=w709:dbl, "Vin / Vout 4"=w720:dbl, "Vin / Vout 5"=w708:dbl, "Manual Gain 1"=w714:dbl, "Manual Gain 2"=w716:dbl, "Manual Gain 3"=w717:dbl)
        n615 = Multiply(x=w744, y=w721) -> (x*y=w743:dbl)
        n616 = Multiply(x=w742, y=w709) -> (x*y=w741:dbl)
        n617 = Divide(x=w754, y=w715) -> (x/y=w750:dbl)
        n618 = Divide(x=w755, y=w718) -> (x/y=w749:dbl)
        n619 = Divide(x=w748, y=w713) -> (x/y=w747:dbl)
        n620 = Divide(x=w745, y=w711) -> (x/y=w746:dbl)
        n621 = Divide(x=w757, y=w719) -> (x/y=w751:dbl)
        n622 = Multiply(x=w750, y=w716) -> (x*y=w726:dbl)
        n623 = Multiply(x=w749, y=w717) -> (x*y=w738:dbl)
        n624 = Multiply(x=w723, y=w759) -> (x*y=w758:dbl)
        n625 = Multiply(x=w743, y=w720) -> (x*y=w732:dbl)
        "V_backgate [V]" <- w732
        n626 = Multiply(x=w741, y=w708) -> (x*y=w730:dbl)
        "V_topgate [V]" <- w730
        n627 = Multiply(x=w747, y=w712) -> (x*y=w734:dbl)
        "Vxx [V]" <- w734
        n628 = Multiply(x=w746, y=w710) -> (x*y=w691:dbl)
        "Vxy [V]" <- w691
        n629 = Multiply(x=w751, y=w714) -> (x*y=w689:dbl)
        n630 = Multiply(x=w726, y=1000000000.0) -> (x*y=w725:dbl)
        "I Leak BG [nA]" <- w725
        n631 = Multiply(x=w738, y=1000000000.0) -> (x*y=w729:dbl)
        "I Leak TG[nA]" <- w729
        n632 = Multiply(x=w758, y=w722) -> (x*y=w740:dbl)
        "Vsd [V]" <- w740
        n633 = Multiply(x=w689, y=1000000000.0) -> (x*y=w690:dbl)
        "I 2probe [nA]" <- w690
        n634 = Divide(x=w734, y=w690) -> (x/y=w694:dbl)
        n635 = Divide(x=w691, y=w689) -> (x/y=w688:dbl)
        n636 = Divide(x=w740, y=w690) -> (x/y=w698:dbl)
        n637 = Divide(x=w688, y=1000.0) -> (x/y=w686:dbl)
        n638 = local read "R4probe array"() -> (w735:dbl[])
        n639 = Multiply(x=w694, y=1000000.0) -> (x*y=w693:dbl)
        "R 4probe [kOhm]" <- w693
        n640 = local read "R2probe array"() -> (w736:dbl[])
        n641 = local read "Vbg array"() -> (w680:dbl[])
        n642 = local read "Rxy Array"() -> (w692:dbl[])
        n643 = local read "Vsd array"() -> (w682:dbl[])
        n644 = local read "Vtg array"() -> (w679:dbl[])
        n645 = local read "Vxy array"() -> (w731:dbl[])
        n646 = local read "Ibg array"() -> (w737:dbl[])
        n647 = local read "Vxx array"() -> (w733:dbl[])
        n648 = local read "Isd array"() -> (w681:dbl[])
        n649 = local read "Itg array"() -> (w739:dbl[])
        n650 = Multiply(x=w698, y=1000000.0) -> (x*y=w696:dbl)
        "R 2probe [kOhm]" <- w696
        n651 = Build Array (concatenate)(w735, w693) -> (w669:dbl[])
        n652 = local read "Wavelength array"() -> (w683:dbl[])
        n653 = local write "R4probe array"(w669) -> ()
        n654 = Build Array (concatenate)(w682, w740) -> (w678:dbl[])
        n655 = Build Array (concatenate)(w681, w690) -> (w677:dbl[])
        n656 = Build Array (concatenate)(w680, w732) -> (w676:dbl[])
        n657 = Build Array (concatenate)(w679, w730) -> (w675:dbl[])
        n658 = Build Array (concatenate)(w737, w725) -> (w674:dbl[])
        n659 = Build Array (concatenate)(w739, w729) -> (w673:dbl[])
        n660 = Build Array (concatenate)(w733, w734) -> (w672:dbl[])
        n661 = Build Array (concatenate)(w731, w691) -> (w671:dbl[])
        n662 = Build Array (concatenate)(w736, w696) -> (w670:dbl[])
        n663 = Build Array (concatenate)(w692, w686) -> (w668:dbl[])
        n664 = local write "Vsd array"(w678) -> ()
        n665 = local write "R2probe array"(w670) -> ()
        n666 = local write "Vtg array"(w675) -> ()
        n667 = local write "Vbg array"(w676) -> ()
        n668 = local read "T"() -> (w685:dbl[])
        n669 = local read "B"() -> (w684:dbl[])
        n670 = local write "Rxy Array"(w668) -> ()
        n671 = local write "Vxy array"(w671) -> ()
        n672 = local write "Vxx array"(w672) -> ()
        n673 = local write "Isd array"(w677) -> ()
        n674 = local write "Ibg array"(w674) -> ()
        n675 = local write "Itg array"(w673) -> ()
        n676 = Build Array(w685, w684, w683, w678, w677, w676, w675, w674, w673, w672, w671, w670, w669, w668) -> (w661:dbl[][])
        n677 = call "Evalmutlivar.vi"("Variables"=w660, "Matrix data"=w661, "formula"="Formula 3") -> ("error out"=w655:errorcluster, "Y Values"=→"Formula3Array":dbl[])  [unwired: 1 in]
        n678 = call "Evalmutlivar.vi"("Variables"=w660, "Matrix data"=w661, "formula"="Formula 4") -> ("error out"=w654:errorcluster, "Y Values"=→"Formula4Array":dbl[])  [unwired: 1 in]
        n679 = call "Evalmutlivar.vi"("Variables"=w660, "Matrix data"=w661, "formula"="Formula 1") -> ("error out"=w666:errorcluster, "Y Values"=→"Formula1Array":dbl[])  [unwired: 1 in]
        n680 = call "Evalmutlivar.vi"("Variables"=w660, "Matrix data"=w661, "formula"="Formula 2") -> ("error out"=w656:errorcluster, "Y Values"=→"Formula2Array":dbl[])  [unwired: 1 in]
      }
      frame "stop" {
        n681 = local read "refnum out"() -> (w938:refnum<file>)
        n682 = Close File(refnum=w938) -> ()  [unwired: 1 in, 2 out]
      }
    }
    n683 = global read "stopButton.vi" "stopsignal"() -> (w324:bool)
    n684 = local write "stop"(w324) -> ()
    n685 = Unbundle By Name("Device Cluster") -> ("K2400 1"=→"K2400 1":refnum<visa-resource-name>, "K2400_1"=→"K2400_1":bool, "K2400 2"=→"K2400 2":refnum<visa-resource-name>, "K2400_2"=→"K2400_2":bool, "Lockin1"=→"Lockin1":refnum<visa-resource-name>, "Lockin1 present"=→"Lockin1 present":bool, "Lockin2"=→"Lockin2":refnum<visa-resource-name>, "Lockin2 present"=→"Lockin2 present":bool, "TIC"=→"TIC":refnum<visa-resource-name>, "Tcontrol"=→"Tcontrol":string, "DMM1"=→"DMM1":refnum<visa-resource-name>, "DMM1"=→"DMM1":bool, "DMM2"=→"DMM2":refnum<visa-resource-name>, "DMM2"=→"DMM2":bool, "DAC"=→"DAC":refnum<visa-resource-name>, "DAC present"=→"DAC present":bool, "DAC number 1"=→"DAC number 1":u8, "Bfield query"=→"Bfield query":bool, "Wvlen query"=→"Wvlen query":bool, "ITC signal"=→"ITC signal":T1, "DAC number 2"=→"DAC number 2":u8)
    n686 = Or(x=w327, y="stop") -> (x .or. y?=w325:bool)
    "stopMainLoop" <- w325
  }
  n687 = property on="Vsd" class="CmbBox"("Strings[]"=w3) -> ()  [unwired: 2 in, 2 out]
  n688 = property on="I leak BG" class="CmbBox"("Strings[]"=w3) -> ()  [unwired: 2 in, 2 out]
  n689 = property on="I leak TG" class="CmbBox"("Strings[]"=w3) -> ()  [unwired: 2 in, 2 out]
  n690 = property on="Vxx" class="CmbBox"("Strings[]"=w3) -> ()  [unwired: 2 in, 2 out]
  n691 = property on="I 2probe 2" class="CmbBox"("Strings[]"=w3) -> ()  [unwired: 2 in, 2 out]
  n692 = property on="Vxy" class="CmbBox"("Strings[]"=w3) -> ()  [unwired: 2 in, 2 out]
  n693 = property on="Y-Axis 4" class="CmbBox"("Strings[]"=w1) -> ()  [unwired: 2 in, 2 out]
  n694 = property on="X-Axis 4" class="CmbBox"("Strings[]"=w1) -> ()  [unwired: 2 in, 2 out]
  n695 = property on="Y-Axis 1" class="CmbBox"("Strings[]"=w1) -> ()  [unwired: 2 in, 2 out]
  n696 = property on="X-Axis 1" class="CmbBox"("Strings[]"=w1) -> ()  [unwired: 2 in, 2 out]
  n697 = property on="X-Axis 2" class="CmbBox"("Strings[]"=w1) -> ()  [unwired: 2 in, 2 out]
  n698 = property on="Y-Axis 2" class="CmbBox"("Strings[]"=w1) -> ()  [unwired: 2 in, 2 out]
  n699 = property on="X-Axis 3" class="CmbBox"("Strings[]"=w1) -> ()  [unwired: 2 in, 2 out]
  n700 = property on="Y-Axis 3" class="CmbBox"("Strings[]"=w1) -> ()  [unwired: 2 in, 2 out]
